vi "CRYPost Processing Name & Unit.vi"(11 "Step setup":string) -> (0 "Run abble?":bool, 1 "Waveform":T2={"Waveform"={"X0"=0.0, "dX"=0.0, "Y"=[]}, "X data"=1, "Y data"=1, "Y axis"=1, "X unit"="s", "Y unit"="V", "Y dB ref"=1.0, "display Y"=TRUE, "display X"=TRUE, "Overload?"=FALSE, "Test Info"="", "Step No."=0, "Name"="", "protected"=FALSE, "Sqc history"=[], "Signal Channel ID"=0, "Plot Settings"={"Color"=0, "Interpolation"=0, "Point Style"=0, "Line Style"=0, "Point Color"=0, "Line Width"=0, "Bar Plot Style"=0, "Fill To"=0}, "AutoProtect"=FALSE} {"Y dB ref" format="%.1f"; "Y axis" items=["Log", "Lin"]; "Y data" items=["dB", "Lin"]; "X data" items=["dB", "Lin"]}, 2 "Data":T3={"Name"="", "Curve"=[], "X data"=1, "Y data"=1, "Z data"=1, "X axis"=0, "Y axis"=1, "Z axis"=1, "X unit"="Hz", "Y unit"="", "Z unit"="deg.", "X dB ref"=1.0, "Y dB ref"=1.0, "Z dB ref"=1.0, "single val"=FALSE, "protected"=FALSE, "display X"=TRUE, "display Y"=TRUE, "display Z"=TRUE, "Test Info"="", "Step No."=0, "Plot Settings"={"Color"=0, "Interpolation"=0, "Point Style"=0, "Line Style"=0, "Point Color"=0, "Line Width"=0, "Bar Plot Style"=0, "Fill To"=0}, "AutoProtect"=FALSE} {"Z data" items=["dB", "Lin"]; "X data" items=["dB", "Lin"]; "Y data" items=["dB", "Lin"]; "Z dB ref" format="%.1f"; "Z axis" items=["Log", "Lin"]; "X dB ref" format="%.1f"; "X axis" items=["Log", "Lin"]; "Y axis" items=["Log", "Lin"]; "Y dB ref" format="%.1f"; "Curve"."z" format="%.2f"; "Curve"."y" format="%.2f"; "Curve"."x" format="%.2f"}, 3 "Result name and type":T4(array[cluster]), 4 "Result":T1={"Name"="Test for Signal [L]", "Margin"=nan, "unit"="", "Verdict"=FALSE, "Limit"="", "Max/Min"="", "protected"=FALSE, "Step No."=0, "Test Info"="", "AutoProtect"=FALSE} {"Margin" format="%.2f"})   [LabVIEW 2013]
uses:
  Typedef Control/CRYData Cluster.ctl
  Typedef Control/CRYWaveform Cluster.ctl
  Typedef Control/CRYResult Cluster.ctl
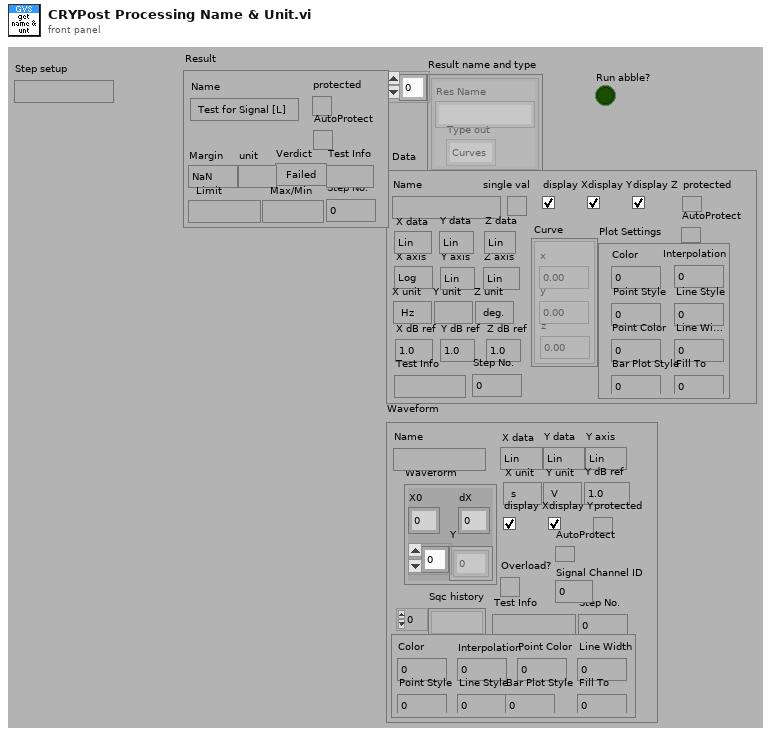
[diagram p1: front panel]
types:
  T1 = typedef "CRYResult Cluster.ctl" = cluster{"Name":string, "Margin":dbl, "unit":string, "Verdict":bool, "Limit":string, "Max/Min":string, "protected":bool, "Step No.":i32, "Test Info":string, "AutoProtect":bool}
  T2 = typedef "CRYWaveform Cluster.ctl" = cluster{"Waveform":cluster{"X0":dbl, "dX":dbl, "Y":sgl[]}, "X data":u16, "Y data":u16, "Y axis":u16, "X unit":string, "Y unit":string, "Y dB ref":dbl, "display Y":bool, "display X":bool, "Overload?":bool, "Test Info":string, "Step No.":i32, "Name":string, "protected":bool, "Sqc history":string[], "Signal Channel ID":i32, "Plot Settings":cluster{"Color":u32, "Interpolation":u8, "Point Style":u8, "Line Style":u8, "Point Color":u32, "Line Width":u8, "Bar Plot Style":u8, "Fill To":i16}, "AutoProtect":bool}
  T3 = typedef "CRYData Cluster.ctl" = cluster{"Name":string, "Curve":cluster{"x":dbl, "y":dbl, "z":dbl}[], "X data":u16, "Y data":u16, "Z data":u16, "X axis":u16, "Y axis":u16, "Z axis":u16, "X unit":string, "Y unit":string, "Z unit":string, "X dB ref":dbl, "Y dB ref":dbl, "Z dB ref":dbl, "single val":bool, "protected":bool, "display X":bool, "display Y":bool, "display Z":bool, "Test Info":string, "Step No.":i32, "Plot Settings":cluster{"Color":u32, "Interpolation":u8, "Point Style":u8, "Line Style":u8, "Point Color":u32, "Line Width":u8, "Bar Plot Style":u8, "Fill To":i16}, "AutoProtect":bool}
  T4 = cluster{"Res Name":string, "Type out":enum16{"Curves", "Values", "Results", "WFM"}}[]
  T5 = cluster{"Type out":enum16{"Curves", "Values", "Results", "WFM"}}[]
  T6 = typedef "CRYPost Processing Cluster.ctl" = cluster{"Name":string, "Op Type":u16, "Curve A":string, "Curve B":string, "Axis Mode":u16, "Work Mode":u16, "Width":u16, "Weighting win":u16, "Search Mode":u16, "Freq Mode":u16, "New Sampling Rate":dbl, "Use Default Name":bool, "x":bool, "y":bool, "z":bool, "All points":bool, "A_single val axis":u16, "B_single val axis":u16, "Use Default Value":bool, "Result Name":string, "Smoothing Width":i32, "Window":u16, "Para_dB":sgl, "Para_%":sgl, "Exponent":sgl, "Hz":dbl, "Direct Weighting":bool, "Auto Inc":bool, "Inc(deg)":i32, "Total Rotation":i32, "Ref Freq Mode":u16, "Ref Waveform":string, "Sampling Rate":dbl, "Weighting Curve":string, "Ref Freq":dbl, "Curve Group":string[], "Search Items":string[], "Custom unit info":cluster{"use custom":bool, "lin/log":u16, "unit":string, "dB ref":dbl, "common dB":u16}, "Unit":string, "Type A":enum16{"Curves", "Values", "Results", "WFM"}, "Type B":enum16{"Curves", "Values", "Results", "WFM"}, "Unary Operator":u16, "Binary Operator":u16, "Statistical Operator":u16, "Constant ":dbl, "New Resolution":u16, "user equation cluster":T7, "Help":string, "Tab Value":enum32{"Setting", "Help"}, "Zwciker_X-axis":u16, "Zwicker_spectrum":bool, "Freq Sampling Mode":u16, "Freq Sampling Rate":dbl, "Smoothing":bool, "Work in Statics":u16, "Result Data":string[]}
  T7 = typedef "CRYUser Equation Cluster.ctl" = cluster{"Custom unit input array":cluster{"use custom":bool, "lin/log":u16, "unit":string, "dB ref":dbl, "common dB":u16}[], "Custom unit results array ":cluster{"use custom":bool, "lin/log":u16, "unit":string, "dB ref":dbl, "common dB":u16}[], "Desired Result Variables":string[], "Desired Result Names":string[], "Input Curve Names":string[], "Input Curve Variables":string[], "equation":string, "Input axis":u16[], "Results axis":u16[], "# input curves":i32, "# Desired result curves ":i32, "Input Values":string[], "Result Values":string[]}
  T8 = enum32{"English", "Chinese", "Korean", "Japanese", "Russian", "Chinese traditional"}
  T9 = cluster{"Res Name":string, "Type out":enum16{"Curves", "Values", "Results", "WFM"}}
  T10 = cluster{"use custom":bool, "lin/log":u16, "unit":string, "dB ref":dbl, "common dB":u16}
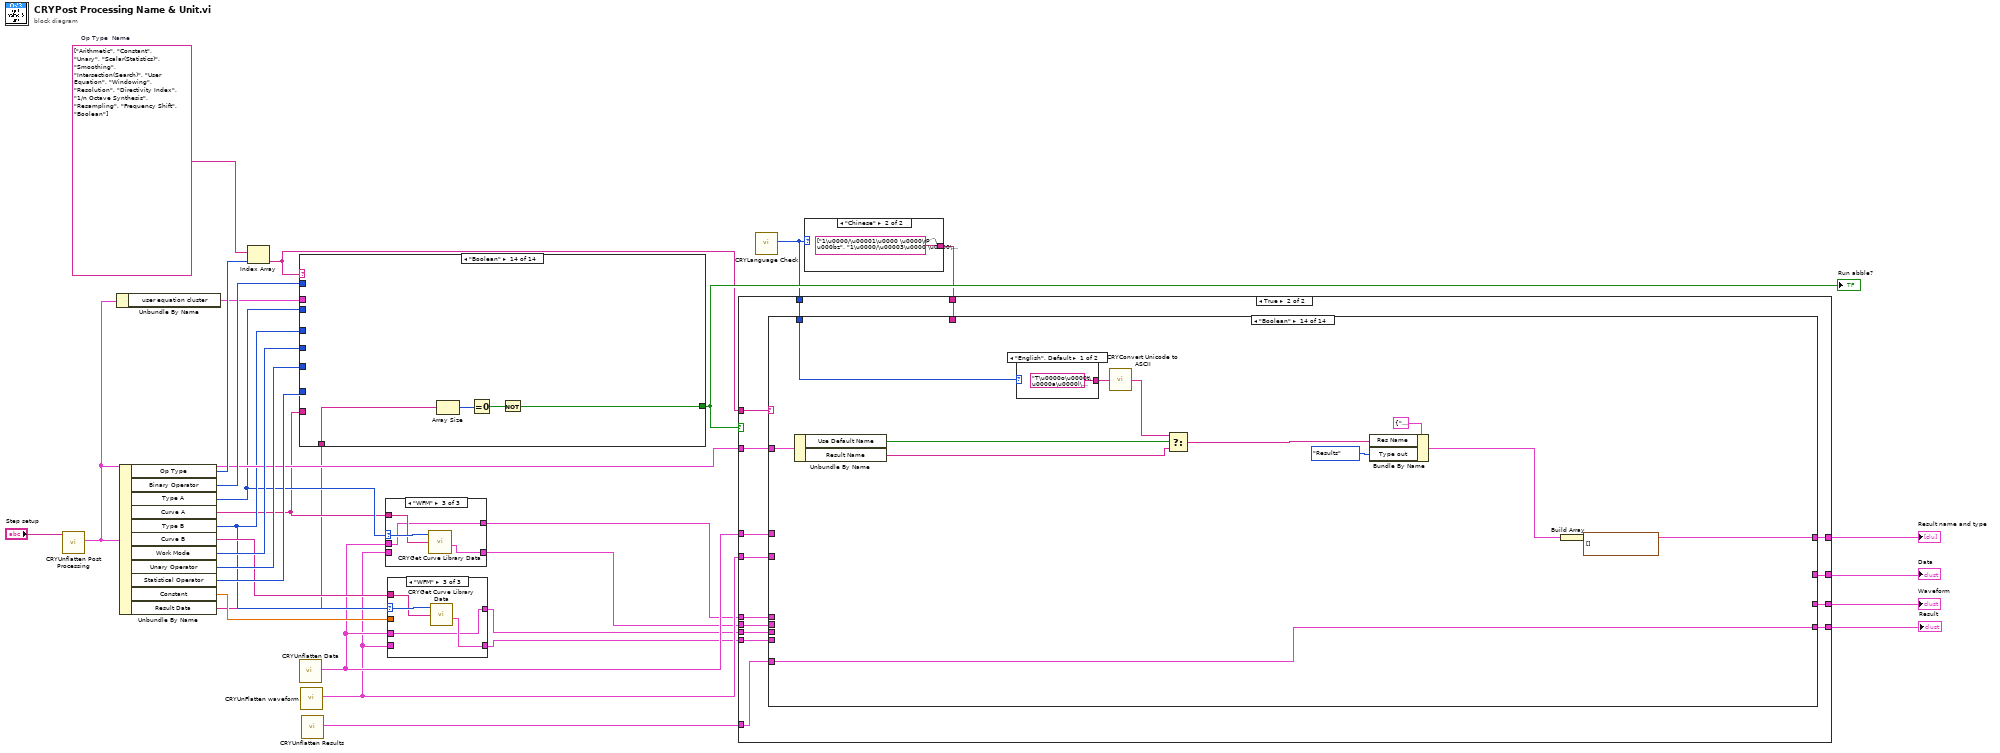
[diagram p0: block diagram]
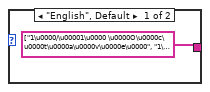
[diagram p2: hidden frame]
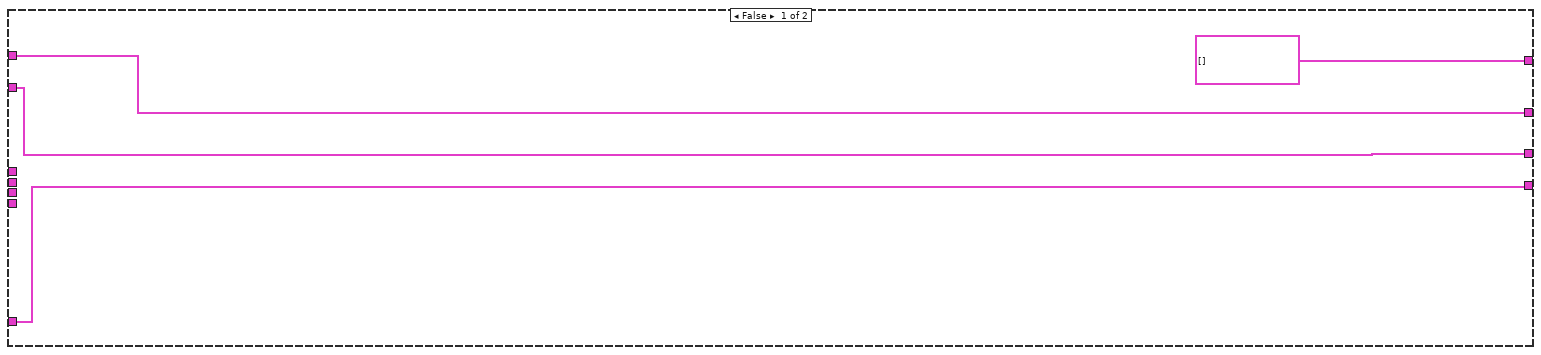
[diagram p3: hidden frame]
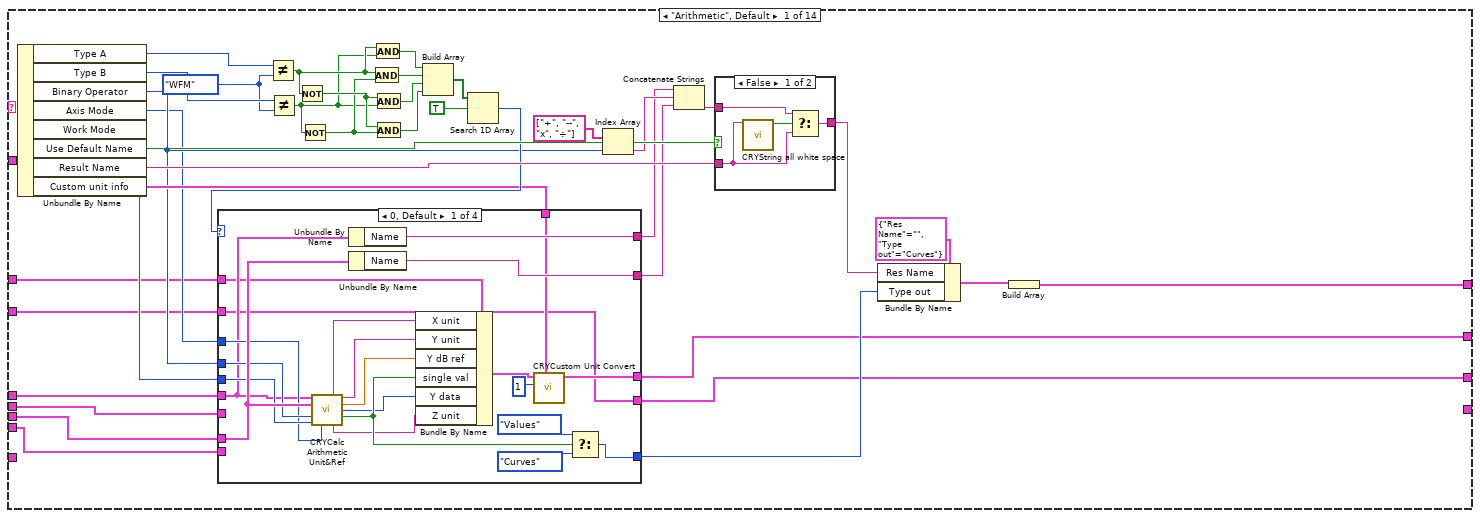
[diagram p4: hidden frame]
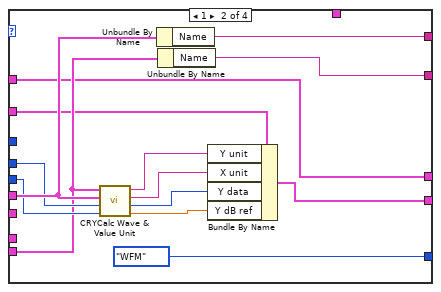
[diagram p5: hidden frame]
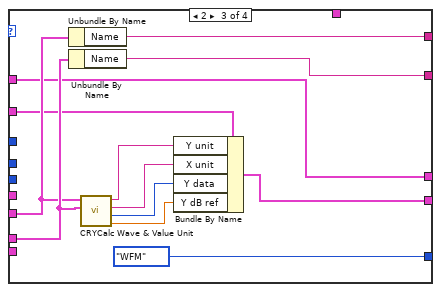
[diagram p6: hidden frame]
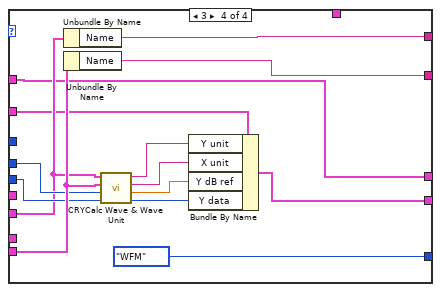
[diagram p7: hidden frame]
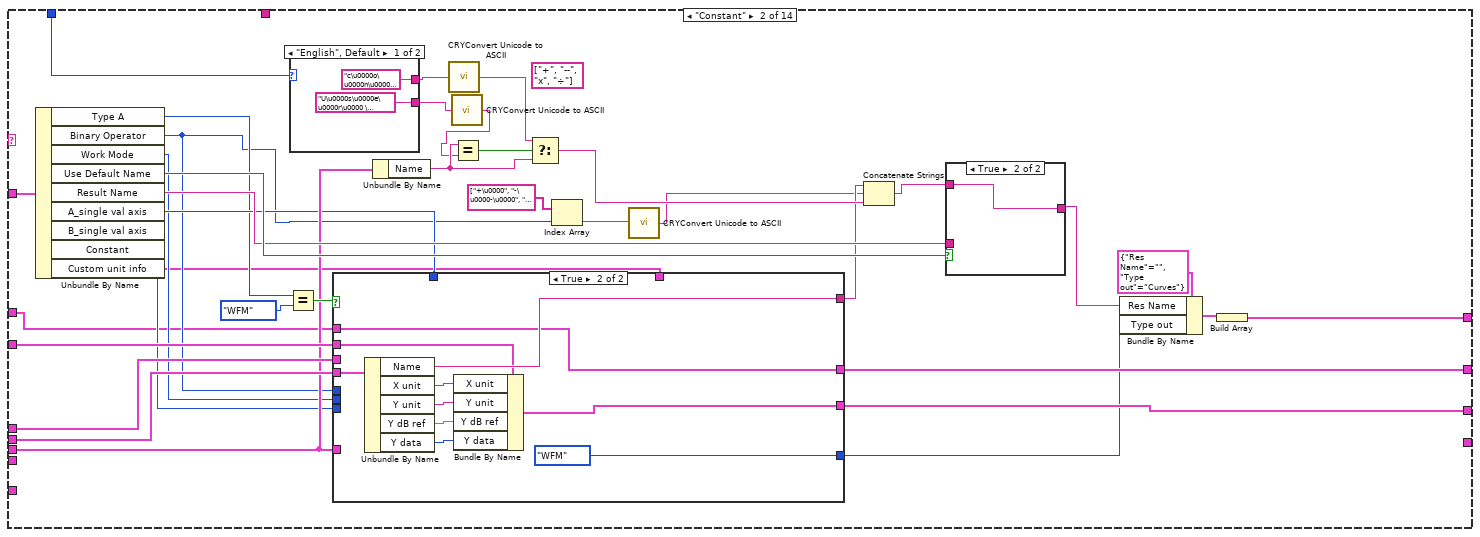
[diagram p9: hidden frame]
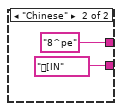
[diagram p10: hidden frame]
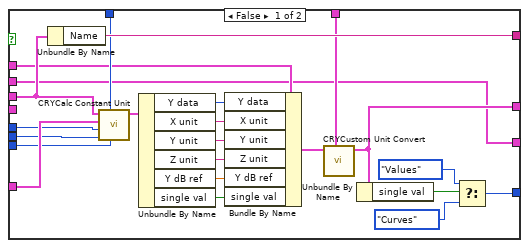
[diagram p11: hidden frame]
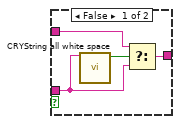
[diagram p12: hidden frame]
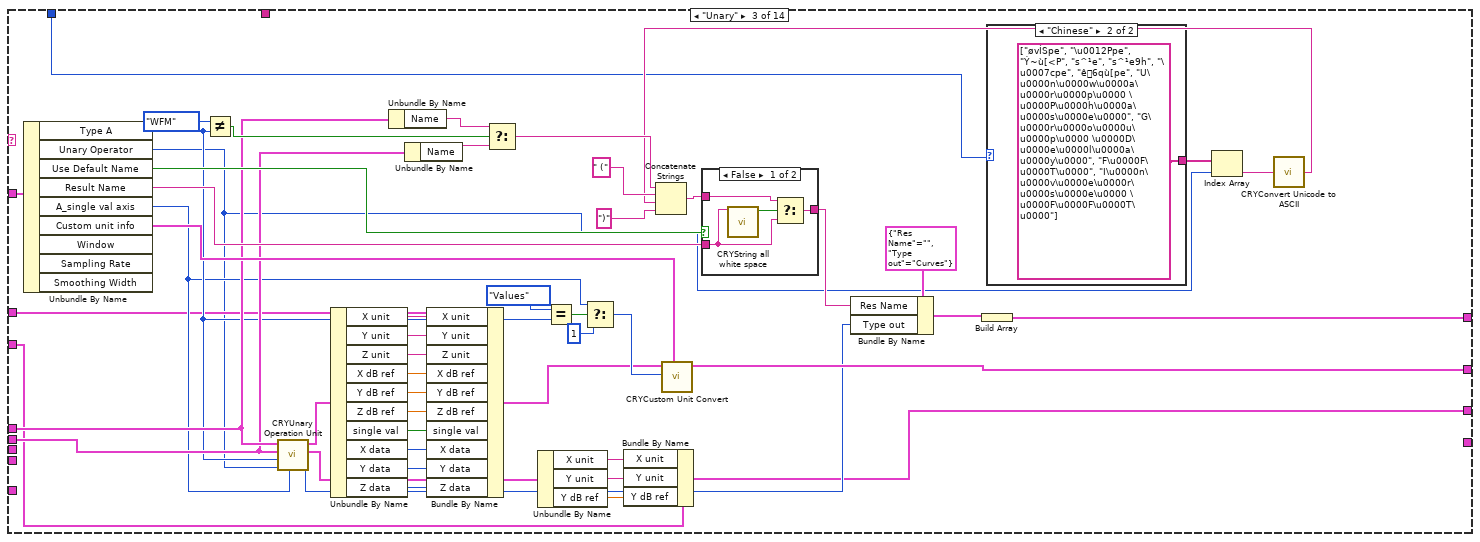
[diagram p13: hidden frame]
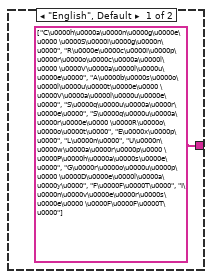
[diagram p14: hidden frame]
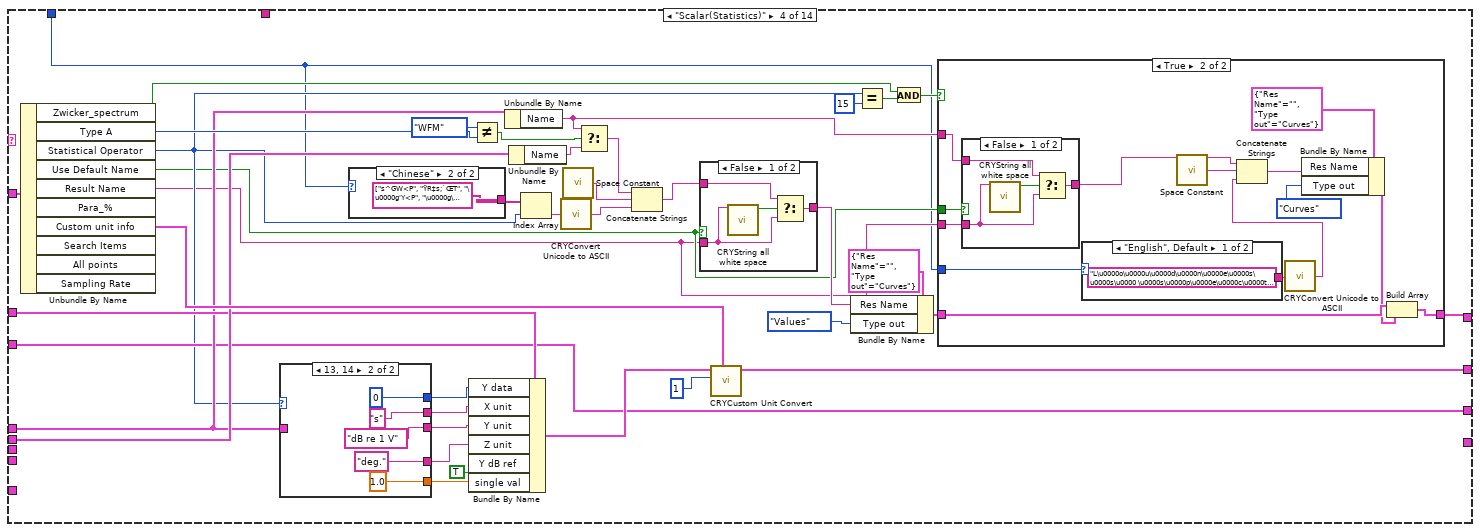
[diagram p16: hidden frame]
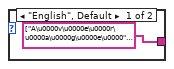
[diagram p17: hidden frame]
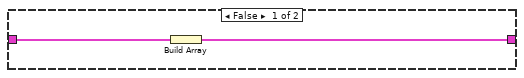
[diagram p18: hidden frame]
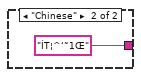
[diagram p19: hidden frame]
diagram:
  (unwired) T5 []
  w30 = string[] ["Arithmetic", "Constant", "Unary", "Scalar(Statistics)", "Smoothing", "Intersection(Search)", "User Equation", "Windowing", "Resolution", "Directivity Index", "1/n Octave Synthesis", "Resampling", "Frequency Shift", "Boolean"]  # Op Type  Name
  n1 = call "CRYUnflatten Post Processing.vi"("Unflatten Post Processing"="Step setup") -> ("Post-Processing"=w18:T6)  [unwired: 10 out]
  n2 = Unbundle By Name(w18) -> ("user equation cluster"=w17:T7)
  n3 = Unbundle By Name(w18) -> ("Op Type"=w27:u16, "Binary Operator"=w26:u16, "Type A"=w13:enum16{"Curves", "Values", "Results", "WFM"}, "Curve A"=w6:string, "Type B"=w14:enum16{"Curves", "Values", "Results", "WFM"}, "Curve B"=w16:string, "Work Mode"=w25:u16, "Unary Operator"=w24:u16, "Statistical Operator"=w23:u16, "Constant"=w15:dbl, "Result Data"=w3:string[])
  n4 = Index Array(array=w30, index=w27) -> (element=w28:string)
  n5 = call "CRYUnflatten Data.vi"() -> ("Datum"=w12:T3)  [unwired: 9 in, 2 out]
  n6 = case shown="\"Boolean\"" w28 {
    tunnel: w13 -> [w34 _ w72 w102 _ w127 _ _ _ _ _ _ _ _]
    tunnel: w14 -> [w33 _ _ _ _ w124 _ _ _ _ _ _ _ _]
    tunnel: w25 -> [w36 w58 _ _ _ _ _ _ _ _ _ _ _ _]
    tunnel: [w31 w55 w67 w100 TRUE w121 TRUE ("x") TRUE TRUE TRUE TRUE w140 w143 w147] -> w29
    tunnel: w24 -> [_ _ w71 _ _ _ _ _ _ _ _ _ _ _]
    tunnel: w23 -> [_ _ _ w98 _ _ _ _ _ _ _ _ _ _]
    tunnel: w26 -> [w35 w57 _ _ _ _ _ _ _ _ _ _ _ _]
    tunnel: w17 -> [_ _ _ _ _ _ _ _ _ _ _ _ _ _]
    tunnel: w6 -> [_ _ _ _ _ _ _ _ _ _ _ w142 w144 _]
    tunnel: w3 -> [_ _ _ _ _ _ _ _ _ _ _ _ _ w146]
    frame "Arithmetic", Default {
      w48 = u16 3 items=["+", "--", "x", "/"] ("Operator")
      w46 = u16 2 items=["+", "--", "x", "/"] ("Operator")
      w45 = u16 0 items=["dB", "Linear", "Power"] ("Work in")
      n7 = Equal?(x=enum16{"Curves", "Values", "Results", "WFM"}."Curves" ("Type A"), y=w34) -> (x = y?=w39:bool)
      n8 = Equal?(x=w33, y=enum16{"Curves", "Values", "Results", "WFM"}."WFM") -> (x = y?=w40:bool)
      n9 = Equal?(x=enum16{"Curves", "Values", "Results", "WFM"}."WFM" ("Type A"), y=w34) -> (x = y?=w43:bool)
      n10 = Equal?(x=w33, y=enum16{"Curves", "Values", "Results", "WFM"}."Curves") -> (x = y?=w44:bool)
      n11 = And(x=w43, y=w44) -> (x .and. y?=w54:bool)
      n12 = And(x=w39, y=w40) -> (x .and. y?=w53:bool)
      n13 = Equal?(x=w36, y=w45) -> (x = y?=w49:bool)
      n14 = Equal?(x=w46, y=w35) -> (x = y?=w47:bool)
      n15 = Equal?(x=w48, y=w35) -> (x = y?=w50:bool)
      n16 = And(x=w49, y=w47) -> (x .and. y?=w51:bool)
      n17 = And(x=w49, y=w50) -> (x .and. y?=w52:bool)
      n18 = Compound Arithmetic op=OR(w51, w52, w53, w54) -> (w32:bool)
      n19 = Not(x=w32) -> (.not. x?=w31:bool)
    }
    frame "Constant" {
      w62 = u16 3 items=["+", "--", "x", "/"] ("Operator")
      w60 = u16 2 items=["+", "--", "x", "/"] ("Operator")
      w59 = u16 0 items=["dB", "Linear", "Power"] ("Work in")
      n20 = Equal?(x=w58, y=w59) -> (x = y?=w63:bool)
      n21 = Equal?(x=w60, y=w57) -> (x = y?=w61:bool)
      n22 = Equal?(x=w62, y=w57) -> (x = y?=w64:bool)
      n23 = And(x=w63, y=w61) -> (x .and. y?=w66:bool)
      n24 = And(x=w63, y=w64) -> (x .and. y?=w65:bool)
      n25 = Or(x=w66, y=w65) -> (x .or. y?=w56:bool)
      n26 = Not(x=w56) -> (.not. x?=w55:bool)
    }
    frame "Unary" {
      n27 = Equal?(x=enum16{"Curves", "Values", "Results", "WFM"}."Curves", y=w72) -> (x = y?=w75:bool)
      n28 = Equal?(x=u16 9, y=w71) -> (x = y?=w77:bool)
      n29 = And(x=w75, y=w77) -> (x .and. y?=w86:bool)
      n30 = Equal?(x=w71, y=u16 7) -> (x = y?=w83:bool)
      n31 = Equal?(x=w71, y=u16 8) -> (x = y?=w84:bool)
      n32 = Equal?(x=w71, y=u16 10) -> (x = y?=w85:bool)
      n33 = Equal?(x=enum16{"Curves", "Values", "Results", "WFM"}."Values", y=w72) -> (x = y?=w94:bool)
      n34 = Equal?(x=enum16{"Curves", "Values", "Results", "WFM"}."WFM", y=w72) -> (x = y?=w82:bool)
      n35 = And(x=w94, y=w77) -> (x .and. y?=w87:bool)
      n36 = And(x=w82, y=w83) -> (x .and. y?=w88:bool)
      n37 = And(x=w82, y=w84) -> (x .and. y?=w89:bool)
      n38 = And(x=w82, y=w85) -> (x .and. y?=w90:bool)
      n39 = Compound Arithmetic op=OR(w86, w87, w88, w89, w90) -> (w69:bool)
      n40 = Equal?(x=w71, y=u16 8) -> (x = y?=w93:bool)
      n41 = Equal?(x=w71, y=u16 10) -> (x = y?=w95:bool)
      n42 = And(x=w94, y=w93) -> (x .and. y?=w96:bool)
      n43 = And(x=w94, y=w95) -> (x .and. y?=w97:bool)
      n44 = Or(x=w96, y=w97) -> (x .or. y?=w70:bool)
      n45 = Or(x=w70, y=w69) -> (x .or. y?=w68:bool)
      n46 = Not(x=w68) -> (.not. x?=w67:bool)
    }
    frame "Scalar(Statistics)" {
      n47 = Index Array(array=string[] ["Average", "Power Sum", "Maximum", "Minimum", "Est. Resonance", "Est. Notch", "IEEE TOLR", "IEEE ROLR", "IEEE SOLR", "ITU-T SLR", "ITU-T RLR", "ITU-T RLR w/ Leak", "ITU-T STMR", "Attack Time", "Release Time", "Zwicker Loudness"] ("Scalar Op Name"), index=w98) -> (element=w101:string)
      n48 = case shown="\"IEEE TOLR\"" w101 {
        tunnel: w102 -> [_ w105 w109 w113 w117]
        tunnel: [TRUE w104 w108 w112 w116] -> w100
        frame "Average", "Maximum", "Minimum", "Power Sum", Default {
        }
        frame "Est. Notch", "Est. Resonance" {
          n49 = case shown="\"Curves\", Default" w105 {
            tunnel: [TRUE FALSE ("x")] -> w104
            frame "Curves", Default {
            }
            frame "WFM" {
            }
          }
        }
        frame "Attack Time", "Release Time" {
          n50 = case shown="\"Curves\"" w109 {
            tunnel: [TRUE FALSE] -> w108
            frame "WFM", Default {
            }
            frame "Curves" {
            }
          }
        }
        frame "Zwicker Loudness" {
          n51 = case shown="\"WFM\"" w113 {
            tunnel: [TRUE FALSE] -> w112
            frame "Curves", Default {
            }
            frame "WFM" {
            }
          }
        }
        frame "IEEE TOLR" {
          n52 = case shown="\"WFM\"" w117 {
            tunnel: [TRUE FALSE] -> w116
            frame "Curves", Default {
            }
            frame "WFM" {
            }
          }
        }
      }
    }
    frame "Smoothing" {
    }
    frame "Intersection(Search)" {
      n53 = Equal?(x=w124, y=enum16{"Curves", "Values", "Results", "WFM"}."Curves" ("Type A")) -> (x = y?=w123:bool)
      n54 = Equal?(x=w124, y=enum16{"Curves", "Values", "Results", "WFM"}."WFM" ("Type A")) -> (x = y?=w134:bool)
      n55 = Equal?(x=w127, y=enum16{"Curves", "Values", "Results", "WFM"}."WFM" ("Type A")) -> (x = y?=w133:bool)
      n56 = Equal?(x=w127, y=enum16{"Curves", "Values", "Results", "WFM"}."Curves" ("Type A")) -> (x = y?=w126:bool)
      n57 = And(x=w133, y=w123) -> (x .and. y?=w131:bool)
      n58 = And(x=w126, y=w134) -> (x .and. y?=w132:bool)
      n59 = Or(x=w131, y=w132) -> (x .or. y?=w122:bool)
      n60 = Not(x=w122) -> (.not. x?=w121:bool)
    }
    frame "User Equation" {
    }
    frame "Windowing" {
    }
    frame "Resolution" {
    }
    frame "Directivity Index" {
    }
    frame "1/n Octave Synthesis" {
    }
    frame "Resampling" {
      n61 = Empty String/Path?(string/path=w142) -> (empty?=w141:bool)
      n62 = Not(x=w141) -> (.not. x?=w140:bool)
    }
    frame "Frequency Shift" {
      n63 = Empty String/Path?(string/path=w144) -> (empty?=w145:bool)
      n64 = Not(x=w145) -> (.not. x?=w143:bool)
    }
    frame "Boolean" {
      n65 = Array Size(array=w146) -> (size(s)=w149:i32)
      n66 = Equal To 0?(x=w149) -> (x = 0?=w148:bool)
      n67 = Not(x=w148) -> (.not. x?=w147:bool)
    }
  }
  "Run abble?" <- w29
  n68 = call "CRYUnFlatten waveform.vi"() -> ("Waveform Cluster"=w11:T2)  [unwired: 9 in, 2 out]
  n69 = call "CRYUnflatten Results.vi"() -> ("Result"=w2:T1)  [unwired: 9 in, 2 out]
  n70 = case shown="\"WFM\"" w13 {
    selector: w13 -> [w153 _ w160]
    tunnel: w6 -> [w152 w156 w159]
    tunnel: [w151 w155 w157] -> w10
    tunnel: w11 -> [w150 w154 _]
    tunnel: w12 -> [_ _ w157]
    tunnel: [w150 w154 w158] -> w9
    frame "Curves", Default {
      n71 = call "CRYGet Curve Library Data.vi"("Type"=w153, "Data Name"=w152) -> ("Curve"=w151:T3)  [unwired: 4 out]
    }
    frame "Values" {
      n72 = call "CRYGet Post Constant Value.vi"("Data Name"=w156) -> ("Value"=w155:T3)  [unwired: 2 in, 8 out]
    }
    frame "WFM" {
      n73 = call "CRYGet Curve Library Data.vi"("Type"=w160, "Data Name"=w159) -> ("Wave"=w158:T2)  [unwired: 4 out]
    }
  }
  n74 = case shown="\"WFM\"" w14 {
    selector: w14 -> [w164 _ w172]
    tunnel: w16 -> [w163 w168 w171]
    tunnel: w15 -> [_ w167 _]
    tunnel: w12 -> [_ _ w169]
    tunnel: w11 -> [w161 w165 _]
    tunnel: [w162 w166 w169] -> w8
    tunnel: [w161 w165 w170] -> w7
    frame "Curves", Default {
      n75 = call "CRYGet Curve Library Data.vi"("Type"=w164, "Data Name"=w163) -> ("Curve"=w162:T3)  [unwired: 4 out]
    }
    frame "Values" {
      n76 = call "CRYGet Post Constant Value.vi"("Constant"=w167, "Data Name"=w168) -> ("Value"=w166:T3)  [unwired: 1 in, 8 out]
    }
    frame "WFM" {
      n77 = call "CRYGet Curve Library Data.vi"("Type"=w172, "Data Name"=w171) -> ("Wave"=w170:T2)  [unwired: 4 out]
    }
  }
  n78 = call "CRYLanguage Check.vi"() -> ("Language"=w4:T8)  [unwired: 10 in, 1 out]
  n79 = case shown="\"Chinese\"" w4 {
    tunnel: [string[] ["1\u0000/\u00001\u0000 \u0000O\u0000c\u0000t\u0000a\u0000v\u0000e\u0000", "1\u0000/\u00003\u0000 \u0000O\u0000c\u0000t\u0000a\u0000v\u0000e\u0000", "1\u0000/\u00006\u0000 \u0000O\u0000c\u0000t\u0000a\u0000v\u0000e\u0000", "1\u0000/\u00001\u00002\u0000 \u0000O\u0000c\u0000t\u0000a\u0000v\u0000e\u0000", "1\u0000/\u00002\u00004\u0000 \u0000O\u0000c\u0000t\u0000a\u0000v\u0000e\u0000", "U\u0000s\u0000e\u0000r\u0000 \u0000D\u0000e\u0000f\u0000i\u0000n\u0000e\u0000d\u0000 \u0000l\u0000o\u0000g\u0000", "U\u0000s\u0000e\u0000r\u0000 \u0000D\u0000e\u0000f\u0000i\u0000n\u0000e\u0000d\u0000 \u0000l\u0000i\u0000n\u0000"] string[] ["1\u0000/\u00001\u0000 \u0000\rP‘˜\u000bz", "1\u0000/\u00003\u0000 \u0000\rP‘˜\u000bz", "1\u0000/\u00006\u0000 \u0000\rP‘˜\u000bz", "1\u0000/\u00001\u00002\u0000 \u0000\rP‘˜\u000bz", "1\u0000/\u00002\u00004\u0000 \u0000\rP‘˜\u000bz", "ê[INù[pe", "ê[IN¿~'`"]] -> w5
    frame "English", Default {
    }
    frame "Chinese" {
    }
  }
  n80 = case shown="True" w29 {
    tunnel: w28 -> [_ w193]
    tunnel: w18 -> [_ w192]
    tunnel: w10 -> [_ w191]
    tunnel: w9 -> [_ w190]
    tunnel: w8 -> [_ w189]
    tunnel: w7 -> [_ w188]
    tunnel: w11 -> [w177 w187]
    tunnel: w12 -> [w176 w186]
    tunnel: [T4 [] w185] -> w21
    tunnel: [w176 w184] -> w20
    tunnel: [w177 w183] -> w19
    tunnel: w5 -> [_ w182]
    tunnel: w4 -> [_ w181]
    tunnel: w2 -> [w175 w180]
    tunnel: [w175 w179] -> w1
    frame False {
    }
    frame True {
      n81 = case shown="\"Boolean\"" w193 {
        tunnel: w192 -> [w232 w332 w424 w472 w548 w641 w704 w726 w794 w851 w891 w921 w959 w983]
        tunnel: w191 -> [w208 w321 w406 w452 w547 w616 _ w715 w779 w838 w878 _ _ _]
        tunnel: w190 -> [w207 w322 w405 w467 w538 w612 _ w711 _ _ _ w914 w945 _]
        tunnel: w189 -> [w206 w316 _ _ _ w613 _ _ _ _ _ _ _ _]
        tunnel: w188 -> [w205 _ _ _ _ w609 _ _ _ _ _ _ _ _]
        tunnel: [w197 w317 w416 w450 w540 w626 w699 w713 w776 w834 w880 w907 w951 _] -> w184
        tunnel: [w196 w318 w395 w448 w537 w610 w698 w712 w775 w833 w869 w908 w943 _] -> w183
        tunnel: [w224 w325 w407 w446 w532 w621 w700 w719 w788 w846 w882 w915 w950 w980] -> w185
        tunnel: w187 -> [w194 w319 w399 w448 w531 w610 w698 w710 w775 w833 w869 w913 w944 _]
        tunnel: w186 -> [w195 w310 w394 w458 w530 w615 w699 w714 w778 w837 w877 w907 w942 _]
        tunnel: w182 -> [_ _ _ _ w516 _ _ _ w763 _ w868 _ _ _]
        tunnel: w181 -> [_ w303 w378 w435 w515 w602 _ _ w762 w830 w865 w906 w937 w978]
        tunnel: w180 -> [_ _ _ _ _ _ _ _ _ _ _ _ _ w974]
        tunnel: [_ _ _ _ _ _ _ _ _ _ _ _ _ w974] -> w179
        frame "Arithmetic", Default {
          w199 = enum16{"Curves", "Values", "Results", "WFM"}."WFM" ("Type A")
          n82 = Unbundle By Name(w232) -> ("Type A"=w212:enum16{"Curves", "Values", "Results", "WFM"}, "Type B"=w211:enum16{"Curves", "Values", "Results", "WFM"}, "Binary Operator"=w202:u16, "Axis Mode"=w200:u16, "Work Mode"=w201:u16, "Use Default Name"=w230:bool, "Result Name"=w229:string, "Custom unit info"=w209:T10)
          n83 = Not Equal?(x=w212, y=w199) -> (x != y?=w219:bool)
          n84 = Not Equal?(x=w211, y=w199) -> (x != y?=w216:bool)
          n85 = Not(x=w219) -> (.not. x?=w218:bool)
          n86 = Not(x=w216) -> (.not. x?=w217:bool)
          n87 = And(x=w219, y=w217) -> (x .and. y?=w215:bool)
          n88 = And(x=w219, y=w216) -> (x .and. y?=w222:bool)
          n89 = And(x=w218, y=w216) -> (x .and. y?=w214:bool)
          n90 = And(x=w218, y=w217) -> (x .and. y?=w213:bool)
          n91 = Build Array(w222, w215, w214, w213) -> (w221:bool[])
          n92 = Search 1D Array(1D array=w221, element=TRUE) -> (index of element=w210:i32)  [unwired: 1 out]
          n93 = case shown="0, Default" w210 {
            tunnel: w208 -> [w245 w265 _ _]
            tunnel: w207 -> [_ _ w276 w288]
            tunnel: w206 -> [w249 _ w277 _]
            tunnel: w205 -> [_ w262 _ w291]
            tunnel: [w238 enum16{"Curves", "Values", "Results", "WFM"}."WFM" ("Type In") enum16{"Curves", "Values", "Results", "WFM"}."WFM" ("Type In") enum16{"Curves", "Values", "Results", "WFM"}."WFM" ("Type In")] -> w198
            tunnel: [w254 w268 w280 w294] -> w204
            tunnel: [w253 w267 w279 w293] -> w203
            tunnel: w209 -> [w252 _ _ _]
            tunnel: [w233 w260 w274 w286] -> w196
            tunnel: [w251 w255 w269 w281] -> w197
            tunnel: w202 -> [w248 w264 _ w290]
            tunnel: w201 -> [w247 w263 _ w289]
            tunnel: w200 -> [w246 _ _ _]
            tunnel: w195 -> [w237 w255 w269 w281]
            tunnel: w194 -> [w233 w259 w273 w285]
            frame 0, Default {
              n94 = call "CRYCalc Arithmetic Unit&Ref.vi"("A data for units"=w245, "B data for units"=w249, "operator"=w248, "Work in"=w247, "Axis Mode"=w246) -> ("Result X unit"=w236:string, "Result Y unit"=w244:string, "Result dB ref(A)"=w243:dbl, "Result Y data"=w235:u16, "Single val out"=w241:bool, "Result Z unit"=w234:string)  [unwired: 5 in]
              n95 = Unbundle By Name(w245) -> ("Name"=w254:string)
              n96 = Unbundle By Name(w249) -> ("Name"=w253:string)
              n97 = Bundle By Name(cluster=w237, "X unit"=w236, "Y unit"=w244, "Y dB ref"=w243, "single val"=w241, "Y data"=w235, "Z unit"=w234) -> (w242:T3)
              n98 = call "CRYCustom Unit Convert.vi"("Custom unit info"=w252, "Axis Mode"=u16 1, "Data in"=w242) -> ("Data out"=w251:T3)  [unwired: 8 out]
              n99 = Select(t=enum16{"Curves", "Values", "Results", "WFM"}."Values", s=w241, f=enum16{"Curves", "Values", "Results", "WFM"}."Curves" ("Type In")) -> (s? t:f=w238:enum16{"Curves", "Values", "Results", "WFM"})
            }
            frame 1 {
              n100 = call "CRYCalc Wave & Value Unit.vi"("Work in"=w263, "Operator"=w264, "Value in"=w265, "Wave in"=w262) -> ("Y dB ref"=w256:dbl, "Y data"=w257:u16, "X unit"=w258:string, "Y unit"=w261:string)  [unwired: 4 in]
              n101 = Unbundle By Name(w265) -> ("Name"=w268:string)
              n102 = Unbundle By Name(w262) -> ("Name"=w267:string)
              n103 = Bundle By Name(cluster=w259, "Y unit"=w261, "X unit"=w258, "Y data"=w257, "Y dB ref"=w256) -> (w260:T2)
            }
            frame 2 {
              n104 = Unbundle By Name(w276) -> ("Name"=w280:string)
              n105 = Unbundle By Name(w277) -> ("Name"=w279:string)
              n106 = call "CRYCalc Wave & Value Unit.vi"("Value in"=w277, "Wave in"=w276) -> ("Y dB ref"=w270:dbl, "Y data"=w271:u16, "X unit"=w272:string, "Y unit"=w275:string)  [unwired: 6 in]
              n107 = Bundle By Name(cluster=w273, "Y unit"=w275, "X unit"=w272, "Y data"=w271, "Y dB ref"=w270) -> (w274:T2)
            }
            frame 3 {
              n108 = Unbundle By Name(w288) -> ("Name"=w294:string)
              n109 = Unbundle By Name(w291) -> ("Name"=w293:string)
              n110 = call "CRYCalc Wave & Wave Unit.vi"("Work in"=w289, "Operator"=w290, "Wave in_2"=w291, "Wave in_1"=w288) -> ("Y data"=w282:u16, "Y dB ref"=w283:dbl, "X unit"=w284:string, "Y unit"=w287:string)  [unwired: 4 in]
              n111 = Bundle By Name(cluster=w285, "Y unit"=w287, "X unit"=w284, "Y dB ref"=w283, "Y data"=w282) -> (w286:T2)
            }
          }
          n112 = Index Array(array=string[] ["+", "--", "x", "÷"] ("Arith Op Name"), index=w202) -> (element=w228:string)
          n113 = Concatenate Strings(w204, w228, w203) -> (w231:string)
          n114 = case shown="False" w230 {
            tunnel: w229 -> [w296 _]
            tunnel: w231 -> [w297 w299]
            tunnel: [w295 w299] -> w226
            frame False {
              n115 = call "CRYString all white space.vi"("String"=w296) -> ("Nothing but white space?"=w298:bool)  [unwired: 10 out]
              n116 = Select(t=w297, s=w298, f=w296) -> (s? t:f=w295:string)
            }
            frame True {
            }
          }
          n117 = Bundle By Name(cluster=T9 {"Res Name"="", "Type out"=enum."Curves"} ("output cluster"), "Res Name"=w226, "Type out"=w198) -> (w223:T9)
          n118 = Build Array(w223) -> (w224:T4)
        }
        frame "Constant" {
          (unwired) string[] ["+", "--", "x", "÷"] ("Arith Op Name")
          n119 = Unbundle By Name(w332) -> ("Type A"=w313:enum16{"Curves", "Values", "Results", "WFM"}, "Binary Operator"=w311:u16, "Work Mode"=w312:u16, "Use Default Name"=w334:bool, "Result Name"=w333:string, "A_single val axis"=w315:u16, "B_single val axis"=w314:u16, "Custom unit info"=w309:T10)  [unwired: 1 out]
          n120 = Equal?(x=w313, y=enum16{"Curves", "Values", "Results", "WFM"}."WFM" ("Type A")) -> (x = y?=w323:bool)
          n121 = case shown="\"English\", Default" w303 {
            tunnel: ["c\u0000o\u0000n\u0000s\u0000t\u0000" "8^pe"] -> w307
            tunnel: ["U\u0000s\u0000e\u0000r\u0000 \u0000D\u0000e\u0000f\u0000i\u0000n\u0000e\u0000d\u0000" "ꁚ[IN"] -> w306
            frame "English", Default {
            }
            frame "Chinese" {
            }
          }
          n122 = case shown="True" w323 {
            tunnel: w322 -> [_ w372]
            tunnel: w321 -> [w361 _]
            tunnel: [w362 w371] -> w320
            tunnel: w319 -> [w340 w370]
            tunnel: [w340 w366] -> w318
            tunnel: [w343 w363] -> w317
            tunnel: w316 -> [w360 _]
            tunnel: w315 -> [w359 _]
            tunnel: w314 -> [w358 _]
            tunnel: w312 -> [w357 _]
            tunnel: w311 -> [w356 _]
            tunnel: w310 -> [w354 w363]
            tunnel: w309 -> [w342 _]
            tunnel: [w341 enum16{"Curves", "Values", "Results", "WFM"}."WFM" ("Type In")] -> w308
            frame False {
              n123 = Unbundle By Name(w361) -> ("Name"=w362:string)
              n124 = call "CRYCalc Constant Unit.vi"("B_axis mode"=w358, "A_axis mode"=w359, "Work in"=w357, "Operator"=w356, "B data for units"=w360, "A data for units"=w361) -> ("Result out"=w355:T3)  [unwired: 5 in]
              n125 = Unbundle By Name(w355) -> ("Y data"=w353:u16, "X unit"=w352:string, "Y unit"=w351:string, "Z unit"=w350:string, "Y dB ref"=w349:dbl, "single val"=w348:bool)
              n126 = Bundle By Name(cluster=w354, "Y data"=w353, "X unit"=w352, "Y unit"=w351, "Z unit"=w350, "Y dB ref"=w349, "single val"=w348) -> (w345:T3)
              n127 = call "CRYCustom Unit Convert.vi"("Custom unit info"=w342, "Data in"=w345) -> ("Data out"=w343:T3)  [unwired: 1 in, 8 out]
              n128 = Unbundle By Name(w343) -> ("single val"=w346:bool)
              n129 = Select(t=enum16{"Curves", "Values", "Results", "WFM"}."Values", s=w346, f=enum16{"Curves", "Values", "Results", "WFM"}."Curves" ("Type In")) -> (s? t:f=w341:enum16{"Curves", "Values", "Results", "WFM"})
            }
            frame True {
              n130 = Unbundle By Name(w372) -> ("Name"=w371:string, "X unit"=w369:string, "Y unit"=w368:string, "Y dB ref"=w367:dbl, "Y data"=w365:u16)
              n131 = Bundle By Name(cluster=w370, "X unit"=w369, "Y unit"=w368, "Y dB ref"=w367, "Y data"=w365) -> (w366:T2)
            }
          }
          n132 = Unbundle By Name(w316) -> ("Name"=w329:string)
          n133 = call "CRYConvert Unicode to ASCII.vi"("Unicode"=w307) -> ("ASCII"=w305:string)  [unwired: 4 in]
          n134 = call "CRYConvert Unicode to ASCII.vi"("Unicode"=w306) -> ("ASCII"=w304:string)  [unwired: 4 in]
          n135 = Equal?(x=w329, y=w304) -> (x = y?=w331:bool)
          n136 = Select(t=w305, s=w331, f=w329) -> (s? t:f=w330:string)
          n137 = Index Array(array=string[] ["+\u0000", "-\u0000-\u0000", "x\u0000", "/\u0000\u0000"], index=w311) -> (element=w301:string)
          n138 = call "CRYConvert Unicode to ASCII.vi"("Unicode"=w301) -> ("ASCII"=w300:string)  [unwired: 4 in]
          n139 = Concatenate Strings(w320, w300, w330) -> (w335:string)
          n140 = case shown="True" w334 {
            tunnel: w333 -> [w374 _]
            tunnel: w335 -> [w375 w377]
            tunnel: [w373 w377] -> w326
            frame False {
              n141 = call "CRYString all white space.vi"("String"=w374) -> ("Nothing but white space?"=w376:bool)  [unwired: 10 out]
              n142 = Select(t=w375, s=w376, f=w374) -> (s? t:f=w373:string)
            }
            frame True {
            }
          }
          n143 = Bundle By Name(cluster=T9 {"Res Name"="", "Type out"=enum."Curves"} ("output cluster"), "Res Name"=w326, "Type out"=w308) -> (w327:T9)
          n144 = Build Array(w327) -> (w325:T4)
        }
        frame "Unary" {
          n145 = Unbundle By Name(w424) -> ("Type A"=w404:enum16{"Curves", "Values", "Results", "WFM"}, "Unary Operator"=w381:u16, "Use Default Name"=w426:bool, "Result Name"=w425:string, "A_single val axis"=w403:u16, "Custom unit info"=w421:T10)  [unwired: 3 out]
          n146 = Not Equal?(x=enum16{"Curves", "Values", "Results", "WFM"}."WFM" ("Type In"), y=w404) -> (x != y?=w420:bool)
          n147 = call "CRYUnary Operation Unit.vi"("A _axis mode"=w403, "Unary Operator"=w381, "Type A"=w404, "Wave in"=w405, "Operand A"=w406) -> ("Type out"=w402:enum16{"Curves", "Values", "Results", "WFM"}, "Wave out"=w400:T2, "Result"=w401:T3)  [unwired: 4 in]
          n148 = Unbundle By Name(w401) -> ("X unit"=w393:string, "Y unit"=w392:string, "Z unit"=w391:string, "X dB ref"=w390:dbl, "Y dB ref"=w389:dbl, "Z dB ref"=w388:dbl, "single val"=w387:bool, "X data"=w386:u16, "Y data"=w385:u16, "Z data"=w384:u16)
          n149 = Unbundle By Name(w406) -> ("Name"=w418:string)
          n150 = Unbundle By Name(w405) -> ("Name"=w417:string)
          n151 = Bundle By Name(cluster=w394, "X unit"=w393, "Y unit"=w392, "Z unit"=w391, "X dB ref"=w390, "Y dB ref"=w389, "Z dB ref"=w388, "single val"=w387, "X data"=w386, "Y data"=w385, "Z data"=w384) -> (w383:T3)
          n152 = Select(t=w418, s=w420, f=w417) -> (s? t:f=w419:string)
          n153 = Unbundle By Name(w400) -> ("X unit"=w398:string, "Y unit"=w397:string, "Y dB ref"=w396:dbl)
          n154 = Equal?(x=enum16{"Curves", "Values", "Results", "WFM"}."Values", y=w404) -> (x = y?=w413:bool)
          n155 = Select(t=w403, s=w413, f=u16 1) -> (s? t:f=w411:u16)
          n156 = Bundle By Name(cluster=w399, "X unit"=w398, "Y unit"=w397, "Y dB ref"=w396) -> (w395:T2)
          n157 = call "CRYCustom Unit Convert.vi"("Custom unit info"=w421, "Axis Mode"=w411, "Data in"=w383) -> ("Data out"=w416:T3)  [unwired: 8 out]
          n158 = case shown="\"Chinese\"" w378 {
            tunnel: [string[] ["C\u0000h\u0000a\u0000n\u0000g\u0000e\u0000 \u0000S\u0000i\u0000g\u0000n\u0000", "R\u0000e\u0000c\u0000i\u0000p\u0000r\u0000o\u0000c\u0000a\u0000l\u0000 \u0000V\u0000a\u0000l\u0000u\u0000e\u0000", "A\u0000b\u0000s\u0000o\u0000l\u0000u\u0000t\u0000e\u0000 \u0000V\u0000a\u0000l\u0000u\u0000e\u0000", "S\u0000q\u0000u\u0000a\u0000r\u0000e\u0000", "S\u0000q\u0000u\u0000a\u0000r\u0000e\u0000 \u0000R\u0000o\u0000o\u0000t\u0000", "E\u0000x\u0000p\u0000", "L\u0000n\u0000", "U\u0000n\u0000w\u0000a\u0000r\u0000p\u0000 \u0000P\u0000h\u0000a\u0000s\u0000e\u0000", "G\u0000r\u0000o\u0000u\u0000p\u0000 \u0000D\u0000e\u0000l\u0000a\u0000y\u0000", "F\u0000F\u0000T\u0000", "I\u0000n\u0000v\u0000e\u0000r\u0000s\u0000e\u0000 \u0000F\u0000F\u0000T\u0000"] string[] ["øvÍSpe", "\u0012Ppe", "Ý~ù[<P", "s^¹e", "s^¹e9h", "\u0007cpe", "ê6qù[pe", "U\u0000n\u0000w\u0000a\u0000r\u0000p\u0000 \u0000P\u0000h\u0000a\u0000s\u0000e\u0000", "G\u0000r\u0000o\u0000u\u0000p\u0000 \u0000D\u0000e\u0000l\u0000a\u0000y\u0000", "F\u0000F\u0000T\u0000", "I\u0000n\u0000v\u0000e\u0000r\u0000s\u0000e\u0000 \u0000F\u0000F\u0000T\u0000"]] -> w382
            frame "English", Default {
            }
            frame "Chinese" {
            }
          }
          n159 = Index Array(array=w382, index=w381) -> (element=w380:string)
          n160 = call "CRYConvert Unicode to ASCII.vi"("Unicode"=w380) -> ("ASCII"=w379:string)  [unwired: 4 in]
          n161 = Concatenate Strings(w419, " (" ("string"), w379, ")" ("string")) -> (w427:string)
          n162 = case shown="False" w426 {
            tunnel: w425 -> [w431 _]
            tunnel: w427 -> [w432 w434]
            tunnel: [w430 w434] -> w408
            frame False {
              n163 = call "CRYString all white space.vi"("String"=w431) -> ("Nothing but white space?"=w433:bool)  [unwired: 10 out]
              n164 = Select(t=w432, s=w433, f=w431) -> (s? t:f=w430:string)
            }
            frame True {
            }
          }
          n165 = Bundle By Name(cluster=T9 {"Res Name"="", "Type out"=enum."Curves"} ("output cluster"), "Res Name"=w408, "Type out"=w402) -> (w409:T9)
          n166 = Build Array(w409) -> (w407:T4)
        }
        frame "Scalar(Statistics)" {
          n167 = Unbundle By Name(w472) -> ("Zwicker_spectrum"=w441:bool, "Type A"=w468:enum16{"Curves", "Values", "Results", "WFM"}, "Statistical Operator"=w443:u16, "Use Default Name"=w439:bool, "Result Name"=w438:string, "Custom unit info"=w471:T10)  [unwired: 4 out]
          n168 = case shown="13, 14" w443 {
            tunnel: [w503 u16 0 ("y")] -> w457
            tunnel: [w502 "s" ("Res Name")] -> w456
            tunnel: [w501 "dB re 1 V" ("Res Name")] -> w455
            tunnel: [w500 "deg." ("Res Name")] -> w454
            tunnel: [w499 1.0 ("Constant")] -> w453
            tunnel: w452 -> [w504 _]
            frame 0..12, Default {
              n169 = Unbundle By Name(w504) -> ("Y data"=w503:u16, "X unit"=w502:string, "Y unit"=w501:string, "Z unit"=w500:string, "Y dB ref"=w499:dbl)
            }
            frame 13, 14 {
            }
          }
          n170 = case shown="\"Chinese\"" w435 {
            tunnel: [string[] ["A\u0000v\u0000e\u0000r\u0000a\u0000g\u0000e\u0000", "P\u0000o\u0000w\u0000e\u0000r\u0000 \u0000S\u0000u\u0000m\u0000", "M\u0000a\u0000x\u0000i\u0000m\u0000u\u0000m\u0000", "M\u0000i\u0000n\u0000i\u0000m\u0000u\u0000m\u0000", "E\u0000s\u0000t\u0000.\u0000 \u0000R\u0000e\u0000s\u0000o\u0000n\u0000a\u0000n\u0000c\u0000e\u0000", "E\u0000s\u0000t\u0000.\u0000 \u0000N\u0000o\u0000t\u0000c\u0000h\u0000", "I\u0000E\u0000E\u0000E\u0000 \u0000T\u0000O\u0000L\u0000R\u0000", "I\u0000E\u0000E\u0000E\u0000 \u0000R\u0000O\u0000L\u0000R\u0000", "I\u0000E\u0000E\u0000E\u0000 \u0000S\u0000O\u0000L\u0000R\u0000", "I\u0000T\u0000U\u0000-\u0000T\u0000 \u0000S\u0000L\u0000R\u0000", "I\u0000T\u0000U\u0000-\u0000T\u0000 \u0000R\u0000L\u0000R\u0000", "I\u0000T\u0000U\u0000-\u0000T\u0000 \u0000R\u0000L\u0000R\u0000 \u0000w\u0000/\u0000 \u0000L\u0000e\u0000a\u0000k\u0000", "I\u0000T\u0000U\u0000-\u0000T\u0000 \u0000S\u0000T\u0000M\u0000R\u0000", "A\u0000t\u0000t\u0000a\u0000c\u0000k\u0000 \u0000T\u0000i\u0000m\u0000e\u0000", "R\u0000e\u0000l\u0000e\u0000a\u0000s\u0000e\u0000 \u0000T\u0000i\u0000m\u0000e\u0000", "Z\u0000w\u0000i\u0000c\u0000k\u0000e\u0000r\u0000 \u0000L\u0000o\u0000u\u0000d\u0000n\u0000e\u0000s\u0000s\u0000"] string[] ["s^GW<P", "ŸR‡s;`ŒT", "\u0000g'Y<P", "\u0000g\u000f\\<P", "\u0010Œ/c0O—{", "ÍS\u0010Œ/c0O—{", "I\u0000E\u0000E\u0000E\u0000 \u0000T\u0000O\u0000L\u0000R\u0000", "I\u0000E\u0000E\u0000E\u0000 \u0000R\u0000O\u0000L\u0000R\u0000", "I\u0000E\u0000E\u0000E\u0000 \u0000S\u0000O\u0000L\u0000R\u0000", "I\u0000T\u0000U\u0000-\u0000T\u0000 \u0000S\u0000L\u0000R\u0000", "I\u0000T\u0000U\u0000-\u0000T\u0000 \u0000R\u0000L\u0000R\u0000", "I\u0000T\u0000U\u0000-\u0000T\u0000 \u0000R\u0000L\u0000R\u0000 \u0000w\u0000/\u0000 \u0000L\u0000e\u0000a\u0000k\u0000", "I\u0000T\u0000U\u0000-\u0000T\u0000 \u0000S\u0000T\u0000M\u0000R\u0000", "A\u0000t\u0000t\u0000a\u0000c\u0000k\u0000 \u0000T\u0000i\u0000m\u0000e\u0000", "R\u0000e\u0000l\u0000e\u0000a\u0000s\u0000e\u0000 \u0000T\u0000i\u0000m\u0000e\u0000", "Z\u0000w\u0000i\u0000c\u0000k\u0000e\u0000r\u0000 \u0000L\u0000o\u0000u\u0000d\u0000n\u0000e\u0000s\u0000s\u0000"]] -> w470
            frame "English", Default {
            }
            frame "Chinese" {
            }
          }
          n171 = Bundle By Name(cluster=w458, "Y data"=w457, "X unit"=w456, "Y unit"=w455, "Z unit"=w454, "Y dB ref"=w453, "single val"=TRUE) -> (w451:T3)
          n172 = Not Equal?(x=enum16{"Curves", "Values", "Results", "WFM"}."WFM" ("Type In"), y=w468) -> (x != y?=w466:bool)
          n173 = Unbundle By Name(w452) -> ("Name"=w440:string)
          n174 = Unbundle By Name(w467) -> ("Name"=w465:string)
          n175 = Index Array(array=w470, index=w443) -> (element=w437:string)
          n176 = call "CRYConvert Unicode to ASCII.vi"("Unicode"=w437) -> ("ASCII"=w436:string)  [unwired: 4 in]
          n177 = call <vilib>:"Space Constant.vi"() -> ("String"=w463:string)
          n178 = Select(t=w440, s=w466, f=w465) -> (s? t:f=w464:string)
          n179 = Concatenate Strings(w464, w463, w436) -> (w473:string)
          n180 = case shown="False" w439 {
            tunnel: w438 -> [w511 _]
            tunnel: w473 -> [w512 w514]
            tunnel: [w510 w514] -> w459
            frame False {
              n181 = call "CRYString all white space.vi"("String"=w511) -> ("Nothing but white space?"=w513:bool)  [unwired: 10 out]
              n182 = Select(t=w512, s=w513, f=w511) -> (s? t:f=w510:string)
            }
            frame True {
            }
          }
          n183 = call "CRYCustom Unit Convert.vi"("Custom unit info"=w471, "Axis Mode"=u16 1, "Data in"=w451) -> ("Data out"=w450:T3)  [unwired: 8 out]
          n184 = Bundle By Name(cluster=T9 {"Res Name"="", "Type out"=enum."Curves"} ("output cluster"), "Res Name"=w459, "Type out"=enum16{"Curves", "Values", "Results", "WFM"}."Values" ("Type In")) -> (w447:T9)
          n185 = Equal?(x=w443, y=u16 15) -> (x = y?=w444:bool)
          n186 = And(x=w441, y=w444) -> (x .and. y?=w445:bool)
          n187 = case shown="True" w445 {
            tunnel: w447 -> [w477 w488]
            tunnel: [w476 w489] -> w446
            tunnel: w440 -> [_ w484]
            tunnel: w439 -> [_ w486]
            tunnel: w438 -> [_ w485]
            tunnel: w435 -> [_ w478]
            frame False {
              n188 = Build Array(w477) -> (w476:T4)
            }
            frame True {
              n189 = case shown="False" w486 {
                tunnel: w485 -> [w495 _]
                tunnel: w484 -> [w496 w498]
                tunnel: [w494 w498] -> w482
                frame False {
                  n190 = call "CRYString all white space.vi"("String"=w495) -> ("Nothing but white space?"=w497:bool)  [unwired: 10 out]
                  n191 = Select(t=w496, s=w497, f=w495) -> (s? t:f=w494:string)
                }
                frame True {
                }
              }
              n192 = case shown="\"English\", Default" w478 {
                tunnel: ["L\u0000o\u0000u\u0000d\u0000n\u0000e\u0000s\u0000s\u0000 \u0000s\u0000p\u0000e\u0000c\u0000t\u0000r\u0000u\u0000m\u0000" ("string") "ÍT¦^‘˜1Œ" ("string")] -> w480
                frame "English", Default {
                }
                frame "Chinese" {
                }
              }
              n193 = call <vilib>:"Space Constant.vi"() -> ("String"=w483:string)
              n194 = call "CRYConvert Unicode to ASCII.vi"("Unicode"=w480) -> ("ASCII"=w479:string)  [unwired: 4 in]
              n195 = Concatenate Strings(w482, w483, w479) -> (w481:string)
              n196 = Bundle By Name(cluster=T9 {"Res Name"="", "Type out"=enum."Curves"} ("output cluster"), "Res Name"=w481, "Type out"=enum16{"Curves", "Values", "Results", "WFM"}."Curves" ("Type In")) -> (w487:T9)
              n197 = Build Array(w488, w487) -> (w489:T4)
            }
          }
        }
        frame "Smoothing" {
          n198 = Unbundle By Name(w548) -> ("Type A"=w544:enum16{"Curves", "Values", "Results", "WFM"}, "Width"=w528:u16, "Use Default Name"=w550:bool, "Result Name"=w551:string, "Custom unit info"=w546:T10)  [unwired: 2 out]
          n199 = case shown="\"Chinese\"" w515 {
            tunnel: [".\u0000 \u0000S\u0000m\u0000o\u0000o\u0000t\u0000h\u0000i\u0000n\u0000g\u0000" ("string") ".\u0000 \u0000s^Ñn" ("string")] -> w524
            tunnel: ["U\u0000s\u0000e\u0000r\u0000 \u0000D\u0000e\u0000f\u0000i\u0000n\u0000e\u0000d\u0000 \u0000L\u0000o\u0000g\u0000" ("string") "ê[INù[pe" ("string")] -> w523
            tunnel: ["U\u0000s\u0000e\u0000r\u0000 \u0000D\u0000e\u0000f\u0000i\u0000n\u0000e\u0000d\u0000 \u0000L\u0000i\u0000n\u0000" ("string") "ê[IN¿~'`" ("string")] -> w522
            tunnel: [" \u0000S\u0000m\u0000o\u0000o\u0000t\u0000h\u0000i\u0000n\u0000g\u0000" ("string") "s^Ñn" ("string")] -> w521
            frame "English", Default {
            }
            frame "Chinese" {
            }
          }
          n200 = Not Equal?(x=enum16{"Curves", "Values", "Results", "WFM"}."WFM" ("Type In"), y=w544) -> (x != y?=w539:bool)
          n201 = Index Array(array=w516, index=w528) -> (element=w526:string)
          n202 = Index Array(array=string[] ["1/1 Octave", "1/3 Octave", "1/6 Octave", "1/12 Octave", "1/24 Octave", "User Defined log", "User Defined lin"] ("Arith Op Name"), index=w528) -> (element=w527:string)
          n203 = call "CRYConvert Unicode to ASCII.vi"("Unicode"=w526) -> ("ASCII"=w525:string)  [unwired: 4 in]
          n204 = call "CRYConvert Unicode to ASCII.vi"("Unicode"=w524) -> ("ASCII"=w517:string)  [unwired: 4 in]
          n205 = call "CRYConvert Unicode to ASCII.vi"("Unicode"=w523) -> ("ASCII"=w519:string)  [unwired: 4 in]
          n206 = call "CRYConvert Unicode to ASCII.vi"("Unicode"=w522) -> ("ASCII"=w518:string)  [unwired: 4 in]
          n207 = Unbundle By Name(w547) -> ("Name"=w543:string)
          n208 = Unbundle By Name(w538) -> ("Name"=w541:string)
          n209 = call "CRYConvert Unicode to ASCII.vi"("Unicode"=w521) -> ("ASCII"=w520:string)  [unwired: 4 in]
          n210 = case shown="False" w539 {
            tunnel: w547 -> [_ w578]
            tunnel: w546 -> [_ w582]
            tunnel: [w561 w581] -> w540
            tunnel: [enum16{"Curves", "Values", "Results", "WFM"}."WFM" ("Type In") enum16{"Curves", "Values", "Results", "WFM"}."Curves" ("Type In")] -> w533
            tunnel: w538 -> [w568 _]
            tunnel: [w562 w570] -> w537
            tunnel: w531 -> [w567 w570]
            tunnel: w530 -> [w561 w577]
            frame False {
              n211 = Unbundle By Name(w568) -> ("X unit"=w566:string, "Y unit"=w565:string, "Y dB ref"=w564:dbl, "Y data"=w563:u16)
              n212 = Bundle By Name(cluster=w567, "X unit"=w566, "Y unit"=w565, "Y dB ref"=w564, "Y data"=w563) -> (w562:T2)
            }
            frame True {
              n213 = Unbundle By Name(w578) -> ("X unit"=w576:string, "Y unit"=w575:string, "Z unit"=w574:string, "Y data"=w573:u16, "Y dB ref"=w572:dbl)
              n214 = Bundle By Name(cluster=w577, "X unit"=w576, "Y unit"=w575, "Z unit"=w574, "Y data"=w573, "Y dB ref"=w572) -> (w571:T3)
              n215 = call "CRYCustom Unit Convert.vi"("Custom unit info"=w582, "Axis Mode"=u16 1, "Data in"=w571) -> ("Data out"=w581:T3)  [unwired: 8 out]
            }
          }
          n216 = case shown="Default" w527 {
            tunnel: w525 -> [w587 _ _]
            tunnel: [w588 w592 w596] -> w552
            tunnel: w520 -> [_ w590 w594]
            tunnel: w519 -> [_ w589 _]
            tunnel: w518 -> [_ _ w593]
            tunnel: w517 -> [w583 _ _]
            frame Default {
              n217 = Match Pattern(string=w587, regular expression="ave") -> (before substring=w585:string)  [unwired: 4 out]
              n218 = call <vilib>:"Space Constant.vi"() -> ("String"=w584:string)
              n219 = Concatenate Strings(w584, w585, w583) -> (w588:string)
            }
            frame "User Defined log" {
              n220 = call <vilib>:"Space Constant.vi"() -> ("String"=w591:string)
              n221 = Concatenate Strings(w591, w589, w590) -> (w592:string)
            }
            frame "User Defined lin" {
              n222 = call <vilib>:"Space Constant.vi"() -> ("String"=w595:string)
              n223 = Concatenate Strings(w595, w593, w594) -> (w596:string)
            }
          }
          n224 = Select(t=w543, s=w539, f=w541) -> (s? t:f=w542:string)
          n225 = Concatenate Strings(w542, w552) -> (w549:string)
          n226 = case shown="False" w550 {
            tunnel: w551 -> [w598 _]
            tunnel: w549 -> [w599 w601]
            tunnel: [w597 w601] -> w534
            frame False {
              n227 = call "CRYString all white space.vi"("String"=w598) -> ("Nothing but white space?"=w600:bool)  [unwired: 10 out]
              n228 = Select(t=w599, s=w600, f=w598) -> (s? t:f=w597:string)
            }
            frame True {
            }
          }
          n229 = Bundle By Name(cluster=T9 {"Res Name"="", "Type out"=enum."Curves"} ("output cluster"), "Res Name"=w534, "Type out"=w533) -> (w536:T9)
          n230 = Build Array(w536) -> (w532:T4)
        }
        frame "Intersection(Search)" {
          w618 = enum16{"Curves", "Values", "Results", "WFM"}."WFM" ("Type A")
          n231 = Unbundle By Name(w641) -> ("Type A"=w629:enum16{"Curves", "Values", "Results", "WFM"}, "Use Default Name"=w643:bool, "Result Name"=w644:string, "Type B"=w628:enum16{"Curves", "Values", "Results", "WFM"}, "Custom unit info"=w640:T10, "Search Mode"=w627:u16)  [unwired: 2 out]
          n232 = Not Equal?(x=w629, y=w618) -> (x != y?=w636:bool)
          n233 = Not Equal?(x=w628, y=w618) -> (x != y?=w633:bool)
          n234 = Not(x=w636) -> (.not. x?=w635:bool)
          n235 = Not(x=w633) -> (.not. x?=w634:bool)
          n236 = And(x=w636, y=w634) -> (x .and. y?=w632:bool)
          n237 = And(x=w636, y=w633) -> (x .and. y?=w639:bool)
          n238 = And(x=w635, y=w633) -> (x .and. y?=w631:bool)
          n239 = And(x=w635, y=w634) -> (x .and. y?=w630:bool)
          n240 = Build Array(w639, w632, w631, w630) -> (w638:bool[])
          n241 = Search 1D Array(1D array=w638, element=TRUE) -> (index of element=w617:i32)  [unwired: 1 out]
          n242 = case shown="3" w617 {
            tunnel: w616 -> [w654 w666 _ _]
            tunnel: w615 -> [w653 w664 w674 w684]
            tunnel: [w652 w663 w673 w683] -> w614
            tunnel: w613 -> [w651 _ w675 _]
            tunnel: w612 -> [_ _ w671 w686]
            tunnel: w609 -> [_ w661 _ w681]
            tunnel: [w650 w662 w670 w682] -> w608
            tunnel: [w649 w660 w672 w680] -> w607
            frame 0, Default {
              n243 = Unbundle By Name(w654) -> ("Name"=w650:string, "Y data"=w659:u16, "X unit"=w658:string, "Y unit"=w657:string, "Z unit"=w656:string, "Y dB ref"=w655:dbl)
              n244 = Unbundle By Name(w651) -> ("Name"=w649:string)
              n245 = Bundle By Name(cluster=w653, "Y data"=w659, "X unit"=w658, "Y unit"=w657, "Z unit"=w656, "Y dB ref"=w655) -> (w652:T3)
            }
            frame 1 {
              n246 = Unbundle By Name(w666) -> ("Name"=w662:string, "Y data"=w669:u16, "X unit"=w668:string, "Z unit"=w667:string)
              n247 = Unbundle By Name(w661) -> ("Name"=w660:string)
              n248 = Bundle By Name(cluster=w664, "Y data"=w669, "X unit"=w668, "Y unit"="", "Z unit"=w667) -> (w663:T3)
            }
            frame 2 {
              n249 = Unbundle By Name(w675) -> ("Y data"=w679:u16, "X unit"=w678:string, "Z unit"=w677:string, "Name"=w672:string)
              n250 = Unbundle By Name(w671) -> ("Name"=w670:string)
              n251 = Bundle By Name(cluster=w674, "Y data"=w679, "X unit"=w678, "Y unit"="", "Z unit"=w677) -> (w673:T3)
            }
            frame 3 {
              w685 = ""
              n252 = Unbundle By Name(w686) -> ("Name"=w682:string, "Y data"=w688:u16, "X unit"=w687:string)
              n253 = Unbundle By Name(w681) -> ("Name"=w680:string)
              n254 = Bundle By Name(cluster=w684, "X data"=w688, "X unit"=w687, "Y unit"=w685, "Z unit"=w685) -> (w683:T3)
            }
          }
          n255 = case shown="\"English\", Default" w602 {
            tunnel: [" \u0000a\u0000n\u0000d\u0000 \u0000" ("string") " \u0000a\u0000n\u0000d\u0000 \u0000" ("string")] -> w606
            tunnel: [" \u0000I\u0000n\u0000t\u0000e\u0000r\u0000s\u0000e\u0000c\u0000t\u0000i\u0000o\u0000n\u0000" ("string") " \u0000I\u0000n\u0000t\u0000e\u0000r\u0000s\u0000e\u0000c\u0000t\u0000i\u0000o\u0000n\u0000" ("string")] -> w604
            frame "English", Default {
            }
            frame "Chinese" {
            }
          }
          n256 = call "CRYConvert Unicode to ASCII.vi"("Unicode"=w606) -> ("ASCII"=w605:string)  [unwired: 4 in]
          n257 = call "CRYConvert Unicode to ASCII.vi"("Unicode"=w604) -> ("ASCII"=w603:string)  [unwired: 4 in]
          n258 = case shown="0, 1, Default" w627 {
            tunnel: [TRUE ("single val") FALSE ("single val")] -> w620
            tunnel: [enum16{"Curves", "Values", "Results", "WFM"}."Values" ("Type In") enum16{"Curves", "Values", "Results", "WFM"}."Curves" ("Type In")] -> w611
            frame 0, 1, Default {
            }
            frame 2 {
            }
          }
          n259 = Concatenate Strings(w608, w605, w607, w603) -> (w642:string)
          n260 = case shown="True" w643 {
            tunnel: w644 -> [w694 _]
            tunnel: w642 -> [w695 w697]
            tunnel: [w693 w697] -> w622
            frame False {
              n261 = call "CRYString all white space.vi"("String"=w694) -> ("Nothing but white space?"=w696:bool)  [unwired: 10 out]
              n262 = Select(t=w695, s=w696, f=w694) -> (s? t:f=w693:string)
            }
            frame True {
            }
          }
          n263 = Bundle By Name(cluster=w614, "single val"=w620) -> (w619:T3)
          n264 = call "CRYCustom Unit Convert.vi"("Custom unit info"=w640, "Axis Mode"=u16 1, "Data in"=w619) -> ("Data out"=w626:T3)  [unwired: 8 out]
          n265 = Bundle By Name(cluster=T9 {"Res Name"="", "Type out"=enum."Curves"} ("output cluster"), "Res Name"=w622, "Type out"=w611) -> (w623:T9)
          n266 = Build Array(w623) -> (w621:T4)
        }
        frame "User Equation" {
          n267 = Unbundle By Name(w704) -> ("user equation cluster"=w703:T7)
          n268 = Unbundle By Name(w703) -> ("Desired Result Names"=w702:string[])
          n269 = for {
            tunnel: w702 -> [w707] mode=indexing
            tunnel: T9 {"Res Name"="", "Type out"=enum."Curves"} ("output cluster") -> [w708]
            tunnel: [w706] -> w700 mode=indexing
            n270 = Bundle By Name(cluster=w708, "Res Name"=w707, "Type out"=enum16{"Curves", "Values", "Results", "WFM"}."Curves") -> (w706:T9)
          }
        }
        frame "Windowing" {
          n271 = Unbundle By Name(w726) -> ("Type A"=w718:enum16{"Curves", "Values", "Results", "WFM"}, "Use Default Name"=w728:bool, "Result Name"=w729:string, "Search Items"=w723:string[], "Custom unit info"=w709:T10)
          n272 = case shown="\"Curves\", Default" w718 {
            tunnel: [w752 w754] -> w724
            tunnel: w711 -> [_ w753]
            tunnel: w715 -> [w751 _]
            frame "Curves", Default {
              n273 = Unbundle By Name(w751) -> ("Name"=w752:string)
            }
            frame "WFM" {
              n274 = Unbundle By Name(w753) -> ("Name"=w754:string)
            }
          }
          n275 = Equal?(x=w718, y=enum16{"Curves", "Values", "Results", "WFM"}."Curves") -> (x = y?=w716:bool)
          n276 = case shown="False" w716 {
            tunnel: w715 -> [_ w742]
            tunnel: w714 -> [w730 w741]
            tunnel: [w730 w740] -> w713
            tunnel: [w731 w738] -> w712
            tunnel: w711 -> [w733 _]
            tunnel: w710 -> [w732 w738]
            tunnel: w709 -> [_ w739]
            frame False {
              n277 = Unbundle By Name(w733) -> ("X unit"=w737:string, "Y unit"=w736:string, "Y dB ref"=w735:dbl, "Y data"=w734:u16)
              n278 = Bundle By Name(cluster=w732, "X unit"=w737, "Y unit"=w736, "Y dB ref"=w735, "Y data"=w734) -> (w731:T2)
            }
            frame True {
              n279 = Unbundle By Name(w742) -> ("Y data"=w749:u16, "X unit"=w748:string, "Y unit"=w747:string, "Z unit"=w746:string, "Y dB ref"=w745:dbl, "single val"=w744:bool)
              n280 = Bundle By Name(cluster=w741, "Y data"=w749, "X unit"=w748, "Y unit"=w747, "Z unit"=w746, "Y dB ref"=w745, "single val"=w744) -> (w743:T3)
              n281 = call "CRYCustom Unit Convert.vi"("Custom unit info"=w739, "Axis Mode"=u16 1, "Data in"=w743) -> ("Data out"=w740:T3)  [unwired: 8 out]
            }
          }
          n282 = call "CRYString Array To Dotted Stirng.vi"("String Array"=w723) -> ("Comma String"=w725:string)  [unwired: 10 out]
          n283 = Concatenate Strings(w724, w725) -> (w727:string)
          n284 = case shown="False" w728 {
            tunnel: w729 -> [w756 _]
            tunnel: w727 -> [w757 w759]
            tunnel: [w755 w759] -> w720
            frame False {
              n285 = call "CRYString all white space.vi"("String"=w756) -> ("Nothing but white space?"=w758:bool)  [unwired: 10 out]
              n286 = Select(t=w757, s=w758, f=w756) -> (s? t:f=w755:string)
            }
            frame True {
            }
          }
          n287 = Bundle By Name(cluster=T9 {"Res Name"="", "Type out"=enum."Curves"} ("output cluster"), "Res Name"=w720, "Type out"=w718) -> (w721:T9)
          n288 = Build Array(w721) -> (w719:T4)
        }
        frame "Resolution" {
          n289 = Unbundle By Name(w794) -> ("New Resolution"=w770:u16, "Use Default Name"=w797:bool, "Result Name"=w798:string, "Custom unit info"=w777:T10)
          n290 = case shown="\"Chinese\"" w762 {
            tunnel: [".\u0000 \u0000S\u0000m\u0000o\u0000o\u0000t\u0000h\u0000i\u0000n\u0000g\u0000" ("string") ".\u0000 \u0000S\u0000m\u0000o\u0000o\u0000t\u0000h\u0000i\u0000n\u0000g\u0000" ("string")] -> w774
            tunnel: ["U\u0000s\u0000e\u0000r\u0000 \u0000D\u0000e\u0000f\u0000i\u0000n\u0000e\u0000d\u0000 \u0000L\u0000o\u0000g\u0000" ("string") "U\u0000s\u0000e\u0000r\u0000 \u0000D\u0000e\u0000f\u0000i\u0000n\u0000e\u0000d\u0000 \u0000L\u0000o\u0000g\u0000" ("string")] -> w773
            tunnel: ["U\u0000s\u0000e\u0000r\u0000 \u0000D\u0000e\u0000f\u0000i\u0000n\u0000e\u0000d\u0000 \u0000L\u0000i\u0000n\u0000" ("string") "U\u0000s\u0000e\u0000r\u0000 \u0000D\u0000e\u0000f\u0000i\u0000n\u0000e\u0000d\u0000 \u0000L\u0000i\u0000n\u0000" ("string")] -> w772
            tunnel: ["S\u0000m\u0000o\u0000o\u0000t\u0000h\u0000i\u0000n\u0000g\u0000" ("string") "S\u0000m\u0000o\u0000o\u0000t\u0000h\u0000i\u0000n\u0000g\u0000" ("string")] -> w771
            tunnel: ["R\u0000e\u0000s\u0000o\u0000l\u0000u\u0000t\u0000i\u0000o\u0000n\u0000" ("string") "R\u0000e\u0000s\u0000o\u0000l\u0000u\u0000t\u0000i\u0000o\u0000n\u0000" ("string")] -> w765
            frame "English", Default {
            }
            frame "Chinese" {
            }
          }
          n291 = Unbundle By Name(w779) -> ("Y data"=w786:u16, "X unit"=w785:string, "Y unit"=w784:string, "Z unit"=w783:string, "Y dB ref"=w782:dbl, "single val"=w781:bool)
          n292 = Unbundle By Name(w779) -> ("Name"=w796:string)
          n293 = Index Array(array=string[] ["1/1 Octave", "1/3 Octave", "1/6 Octave", "1/12 Octave", "1/24 Octave", "User Defined log", "User Defined lin"] ("Arith Op Name"), index=w770) -> (element=w799:string)
          n294 = Index Array(array=w763, index=w770) -> (element=w761:string)
          n295 = call "CRYConvert Unicode to ASCII.vi"("Unicode"=w774) -> ("ASCII"=w769:string)  [unwired: 4 in]
          n296 = call "CRYConvert Unicode to ASCII.vi"("Unicode"=w773) -> ("ASCII"=w768:string)  [unwired: 4 in]
          n297 = call "CRYConvert Unicode to ASCII.vi"("Unicode"=w772) -> ("ASCII"=w766:string)  [unwired: 4 in]
          n298 = call "CRYConvert Unicode to ASCII.vi"("Unicode"=w771) -> ("ASCII"=w767:string)  [unwired: 4 in]
          n299 = call "CRYConvert Unicode to ASCII.vi"("Unicode"=w765) -> ("ASCII"=w764:string)  [unwired: 4 in]
          n300 = call "CRYConvert Unicode to ASCII.vi"("Unicode"=w761) -> ("ASCII"=w760:string)  [unwired: 4 in]
          n301 = Bundle By Name(cluster=w778, "Y data"=w786, "X unit"=w785, "Y unit"=w784, "Z unit"=w783, "Y dB ref"=w782, "single val"=w781) -> (w780:T3)
          n302 = case shown="Default" w799 {
            tunnel: w760 -> [w815 _ _]
            tunnel: [w816 w820 w824] -> w800
            tunnel: w769 -> [w811 _ _]
            tunnel: w768 -> [_ w818 _]
            tunnel: w767 -> [_ w817 _]
            tunnel: w766 -> [_ _ w822]
            tunnel: w764 -> [_ _ w821]
            frame Default {
              n303 = Match Pattern(string=w815, regular expression="ave") -> (before substring=w813:string)  [unwired: 4 out]
              n304 = call <vilib>:"Space Constant.vi"() -> ("String"=w812:string)
              n305 = Concatenate Strings(w812, w813, w811) -> (w816:string)
            }
            frame "User Defined log" {
              n306 = call <vilib>:"Space Constant.vi"() -> ("String"=w819:string)
              n307 = Concatenate Strings(w819, w818, w817) -> (w820:string)
            }
            frame "User Defined lin" {
              n308 = call <vilib>:"Space Constant.vi"() -> ("String"=w823:string)
              n309 = Concatenate Strings(w823, w822, w821) -> (w824:string)
            }
          }
          n310 = call "CRYCustom Unit Convert.vi"("Custom unit info"=w777, "Axis Mode"=u16 1, "Data in"=w780) -> ("Data out"=w776:T3)  [unwired: 8 out]
          n311 = Concatenate Strings(w796, w800) -> (w795:string)
          n312 = case shown="True" w797 {
            tunnel: w798 -> [w826 _]
            tunnel: w795 -> [w827 w829]
            tunnel: [w825 w829] -> w790
            frame False {
              n313 = call "CRYString all white space.vi"("String"=w826) -> ("Nothing but white space?"=w828:bool)  [unwired: 10 out]
              n314 = Select(t=w827, s=w828, f=w826) -> (s? t:f=w825:string)
            }
            frame True {
            }
          }
          n315 = Bundle By Name(cluster=T9 {"Res Name"="", "Type out"=enum."Curves"} ("output cluster"), "Res Name"=w790, "Type out"=enum16{"Curves", "Values", "Results", "WFM"}."Curves" ("Data type")) -> (w791:T9)
          n316 = Build Array(w791) -> (w788:T4)
        }
        frame "Directivity Index" {
          n317 = Unbundle By Name(w851) -> ("Use Default Name"=w854:bool, "Result Name"=w855:string, "Custom unit info"=w835:T10)
          n318 = case shown="\"English\", Default" w830 {
            tunnel: ["D\u0000I\u0000" "D\u0000I\u0000"] -> w832
            frame "English", Default {
            }
            frame "Chinese" {
            }
          }
          n319 = Unbundle By Name(w838) -> ("Y data"=w844:u16, "X unit"=w843:string, "Y unit"=w842:string, "Z unit"=w841:string, "Y dB ref"=w840:dbl, "single val"=w839:bool)
          n320 = Unbundle By Name(w838) -> ("Name"=w853:string)
          n321 = call "CRYConvert Unicode to ASCII.vi"("Unicode"=w832) -> ("ASCII"=w831:string)  [unwired: 4 in]
          n322 = Bundle By Name(cluster=w837, "Y data"=w844, "X unit"=w843, "Y unit"=w842, "Z unit"=w841, "Y dB ref"=w840, "single val"=w839) -> (w836:T3)
          n323 = Concatenate Strings(w853, w831) -> (w852:string)
          n324 = case shown="False" w854 {
            tunnel: w855 -> [w859 _]
            tunnel: w852 -> [w860 w862]
            tunnel: [w858 w862] -> w848
            frame False {
              n325 = call "CRYString all white space.vi"("String"=w859) -> ("Nothing but white space?"=w861:bool)  [unwired: 10 out]
              n326 = Select(t=w860, s=w861, f=w859) -> (s? t:f=w858:string)
            }
            frame True {
            }
          }
          n327 = call "CRYCustom Unit Convert.vi"("Custom unit info"=w835, "Axis Mode"=u16 1, "Data in"=w836) -> ("Data out"=w834:T3)  [unwired: 8 out]
          n328 = Bundle By Name(cluster=T9 {"Res Name"="", "Type out"=enum."Curves"} ("output cluster"), "Res Name"=w848, "Type out"=enum16{"Curves", "Values", "Results", "WFM"}."Curves" ("Data type")) -> (w849:T9)
          n329 = Build Array(w849) -> (w846:T4)
        }
        frame "1/n Octave Synthesis" {
          n330 = Unbundle By Name(w891) -> ("New Resolution"=w888:u16, "Use Default Name"=w894:bool, "Result Name"=w895:string, "Custom unit info"=w879:T10)
          n331 = Unbundle By Name(w878) -> ("Name"=w893:string)
          n332 = Unbundle By Name(w878) -> ("Y data"=w876:u16, "X unit"=w875:string, "Y unit"=w874:string, "Z unit"=w873:string, "Y dB ref"=w872:dbl, "single val"=w871:bool)
          n333 = Index Array(array=w868, index=w888) -> (element=w867:string)
          n334 = case shown="\"Chinese\"" w865 {
            tunnel: [".\u0000 \u0000S\u0000y\u0000m\u0000t\u0000h\u0000e\u0000s\u0000i\u0000s\u0000" ("string") ".\u0000 \u0000ü~\bT" ("string")] -> w864
            frame "English", Default {
            }
            frame "Chinese" {
            }
          }
          n335 = call "CRYConvert Unicode to ASCII.vi"("Unicode"=w867) -> ("ASCII"=w866:string)  [unwired: 4 in]
          n336 = Bundle By Name(cluster=w877, "Y data"=w876, "X unit"=w875, "Y unit"=w874, "Z unit"=w873, "Y dB ref"=w872, "single val"=w871) -> (w870:T3)
          n337 = call "CRYConvert Unicode to ASCII.vi"("Unicode"=w864) -> ("ASCII"=w863:string)  [unwired: 4 in]
          n338 = Match Pattern(string=w866, regular expression="ave") -> (before substring=w889:string)  [unwired: 4 out]
          n339 = call <vilib>:"Space Constant.vi"() -> ("String"=w887:string)
          n340 = call "CRYCustom Unit Convert.vi"("Custom unit info"=w879, "Axis Mode"=u16 1, "Data in"=w870) -> ("Data out"=w880:T3)  [unwired: 8 out]
          n341 = Concatenate Strings(w887, w889, w863) -> (w896:string)
          n342 = Concatenate Strings(w893, w896) -> (w892:string)
          n343 = case shown="False" w894 {
            tunnel: w895 -> [w900 _]
            tunnel: w892 -> [w901 w903]
            tunnel: [w899 w903] -> w884
            frame False {
              n344 = call "CRYString all white space.vi"("String"=w900) -> ("Nothing but white space?"=w902:bool)  [unwired: 10 out]
              n345 = Select(t=w901, s=w902, f=w900) -> (s? t:f=w899:string)
            }
            frame True {
            }
          }
          n346 = Bundle By Name(cluster=T9 {"Res Name"="", "Type out"=enum."Curves"} ("output cluster"), "Res Name"=w884, "Type out"=enum16{"Curves", "Values", "Results", "WFM"}."Curves" ("Data type")) -> (w885:T9)
          n347 = Build Array(w885) -> (w882:T4)
        }
        frame "Resampling" {
          n348 = Unbundle By Name(w921) -> ("Use Default Name"=w923:bool, "Result Name"=w924:string)  [unwired: 1 out]
          n349 = case shown="\"Chinese\"" w906 {
            tunnel: ["(\u0000R\u0000e\u0000s\u0000a\u0000m\u0000p\u0000l\u0000i\u0000n\u0000g\u0000)\u0000" ("string") "(\u0000͑Ǒ7h)\u0000" ("string")] -> w905
            frame "English", Default {
            }
            frame "Chinese" {
            }
          }
          n350 = Unbundle By Name(w914) -> ("X unit"=w912:string, "Y unit"=w911:string, "Y dB ref"=w910:dbl, "Y data"=w909:u16)
          n351 = Bundle By Name(cluster=w913, "X unit"=w912, "Y unit"=w911, "Y dB ref"=w910, "Y data"=w909) -> (w908:T2)
          n352 = Unbundle By Name(w914) -> ("Name"=w920:string)
          n353 = call "CRYConvert Unicode to ASCII.vi"("Unicode"=w905) -> ("ASCII"=w904:string)  [unwired: 4 in]
          n354 = Concatenate Strings(w920, w904) -> (w922:string)
          n355 = case shown="False" w923 {
            tunnel: w924 -> [w928 _]
            tunnel: w922 -> [w929 w931]
            tunnel: [w927 w931] -> w917
            frame False {
              n356 = call "CRYString all white space.vi"("String"=w928) -> ("Nothing but white space?"=w930:bool)  [unwired: 10 out]
              n357 = Select(t=w929, s=w930, f=w928) -> (s? t:f=w927:string)
            }
            frame True {
            }
          }
          n358 = Bundle By Name(cluster=T9 {"Res Name"="", "Type out"=enum."Curves"} ("output cluster"), "Res Name"=w917, "Type out"=enum16{"Curves", "Values", "Results", "WFM"}."WFM" ("Type In")) -> (w918:T9)
          n359 = Build Array(w918) -> (w915:T4)
        }
        frame "Frequency Shift" {
          w940 = FALSE ("display Y")
          # "++result=Playback sampling rate(Single Value)=zhunque ?"
          n360 = Unbundle By Name(w959) -> ("Use Default Name"=w961:bool, "Result Name"=w962:string)  [unwired: 3 out]
          n361 = case shown="\"Chinese\"" w937 {
            tunnel: ["(\u0000P\u0000l\u0000a\u0000y\u0000b\u0000a\u0000c\u0000k\u0000 \u0000S\u0000a\u0000m\u0000p\u0000l\u0000i\u0000n\u0000g\u0000 \u0000R\u0000a\u0000t\u0000e\u0000)\u0000" ("string") "(\u0000ÞV>eÇ‘7h‡s)\u0000" ("string")] -> w936
            tunnel: ["(\u0000F\u0000r\u0000e\u0000q\u0000u\u0000e\u0000n\u0000c\u0000y\u0000 \u0000S\u0000h\u0000i\u0000f\u0000t\u0000)\u0000" ("string") "(\u0000slbc)\u0000" ("string")] -> w933
            frame "English", Default {
            }
            frame "Chinese" {
            }
          }
          n362 = Unbundle By Name(w945) -> ("X unit"=w949:string, "Y unit"=w948:string, "Y dB ref"=w947:dbl, "Y data"=w946:u16)
          n363 = Unbundle By Name(w945) -> ("Name"=w958:string)
          n364 = Bundle By Name(cluster=w944, "X unit"=w949, "Y unit"=w948, "Y dB ref"=w947, "Y data"=w946) -> (w943:T2)
          n365 = call "CRYConvert Unicode to ASCII.vi"("Unicode"=w933) -> ("ASCII"=w932:string)  [unwired: 4 in]
          n366 = Concatenate Strings(w958, w932) -> (w960:string)
          n367 = call "CRYConvert Unicode to ASCII.vi"("Unicode"=w936) -> ("ASCII"=w935:string)  [unwired: 4 in]
          n368 = case shown="False" w961 {
            tunnel: w962 -> [w968 _]
            tunnel: w960 -> [w969 w971]
            tunnel: [w967 w971] -> w955
            frame False {
              n369 = call "CRYString all white space.vi"("String"=w968) -> ("Nothing but white space?"=w970:bool)  [unwired: 10 out]
              n370 = Select(t=w969, s=w970, f=w968) -> (s? t:f=w967:string)
            }
            frame True {
            }
          }
          n371 = Concatenate Strings(w958, w935) -> (w934:string)
          n372 = Bundle By Name(cluster=w942, "single val"=TRUE, "X unit"="Hz", "display Y"=w940, "display Z"=w940) -> (w951:T3)
          n373 = Bundle By Name(cluster=T9 {"Res Name"="", "Type out"=enum."Curves"} ("output cluster"), "Res Name"=w955, "Type out"=enum16{"Curves", "Values", "Results", "WFM"}."WFM" ("Type In")) -> (w939:T9)
          n374 = Bundle By Name(cluster=T9 {"Res Name"="", "Type out"=enum."Curves"} ("output cluster"), "Res Name"=w934, "Type out"=enum16{"Curves", "Values", "Results", "WFM"}."Values" ("Type In")) -> (w938:T9)
          n375 = Build Array(w938, w939) -> (w950:T4)
        }
        frame "Boolean" {
          n376 = Unbundle By Name(w983) -> ("Use Default Name"=w976:bool, "Result Name"=w972:string)
          n377 = case shown="\"English\", Default" w978 {
            tunnel: ["T\u0000o\u0000t\u0000a\u0000l\u0000 \u0000R\u0000e\u0000s\u0000u\u0000l\u0000t\u0000" ";`Ó~œg"] -> w977
            frame "English", Default {
            }
            frame "Chinese" {
            }
          }
          n378 = call "CRYConvert Unicode to ASCII.vi"("Unicode"=w977) -> ("ASCII"=w973:string)  [unwired: 4 in]
          n379 = Select(t=w973, s=w976, f=w972) -> (s? t:f=w975:string)
          n380 = Bundle By Name(cluster=T9 {"Res Name"="", "Type out"=enum."Curves"} ("output cluster"), "Res Name"=w975, "Type out"=enum16{"Curves", "Values", "Results", "WFM"}."Results" ("Type In")) -> (w979:T9)
          n381 = Build Array(w979) -> (w980:T4)
        }
      }
    }
  }
  "Result name and type" <- w21
  "Data" <- w20
  "Waveform" <- w19
  "Result" <- w1
